vi "上下管柱装配.vi"() -> ()   [LabVIEW 2018]
uses:
  <vilib>/Utility/config.llb/NI_LVConfig.lvlib
  Global_Variable/Global.vi
  Global_Variable/Global1.vi
  Global_Variable/A131258.vi
  <vilib>/addons/database/NI_Database_API.lvlib
  <vilib>/addons/database/Connection.llb/Conn Execute.vi
  <vilib>/addons/database/Recordset.llb/Rec Fetch Recordset Data (R).vi
  <vilib>/addons/database/Connection.llb/DB Tools Open Connec (String).vi
panel:
  out "RIGHTMIN压力":string
  out "RIGHTMAX压力":string
  out "RIGHT位移":string
  out "LEFTMIN压力":string
  out "LEFTMAX压力":string
  out "LEFT位移":string
  out "RESULT":string
  out "PRODUCTID":string
  out "USERID":string
  out "上管柱码":string
  out "产品型号":string
  in  "附加信息 3":string
  in  "设备状态 3":enum16{"设备离线", "设备正常", "设备缺料", "设备故障", "质量报警"}(ring)=enum."质量报警"
  in  "附加信息 2":string
  in  "设备状态 2":enum16{"设备离线", "设备正常", "设备缺料", "设备故障", "质量报警"}(ring)=enum."设备缺料"
  in  "质量报警":bool
  in  "设备缺料":bool
  in  "附加信息":string
  in  "设备状态":enum16{"设备离线", "设备正常", "设备缺料", "设备故障", "质量报警"}(ring)=enum."设备故障"
  in  "设备故障":bool
  out "前序deviceID":string
  out "deviceID":string
  out "CODE_ID":string
  out "联机模式":string
  out "用户权限":string
  out "用户名":string
  in  "报表":string[][](table)=[["mm"], ["mm/s"]]
  in  "判定结果 3":bool[][](array[boolean])=[[TRUE]]
  in  "选项卡控件 2":enum32{"左工位压装曲线", "右工位压装曲线 ", "参数查看"}(tab)
  out "左压装下限":dbl format="%#.2f"
  out "左压装上限":dbl format="%#.2f"
  out "左下限2":dbl format="%#.2f"
  out "左上限2":dbl format="%#.2f"
  out "左下限1":dbl format="%#.2f"
  out "左上限1":dbl format="%#.2f"
  out "压装最大位移(mm)":dbl
  out "判定结果":bool
  out "力位移曲线":cluster{dbl[], dbl[]}[](graph)
  out "位移区间最大压力(KN)":dbl
  out "位移区间最小压力(KN)":dbl
  out "右位移下限":dbl format="%#.2f"
  out "右位移上限":dbl format="%#.2f"
  out "右下限2":dbl format="%#.2f"
  out "右上限2":dbl format="%#.2f"
  out "右下限1":dbl format="%#.2f"
  out "右上限1":dbl format="%#.2f"
  out "压装最大位移(mm) 2":dbl
  out "判定结果 2":bool
  out "力位移曲线 2":cluster{dbl[], dbl[]}[](graph)
  out "位移区间最大压力(KN) 2":dbl
  out "位移区间最小压力(KN) 2":dbl
  in  "删除":bool
  in  "确定":bool
  in  "添加":bool
  in  "退出":bool
  in  "更新":bool
  in  "产品型号":string(combo)
  in  "选项卡控件 3":enum32{"左工位参数", "右工位参数", "产品管理", "用户管理"}(tab)
  in  "左工位坐标轴参数":string[][](table)=[["mm"], ["mm/s"]]
  in  "左工位判定框参数":string[][](table)=[["mm"], ["mm/s"]]
  in  "左工位结果判定参数":string[][](table)=[["mm"], ["mm/s"]]
  in  "右工位结果判定参数":string[][](table)=[["mm"], ["mm/s"]]
  in  "右工位判定框参数":string[][](table)=[["mm"], ["mm/s"]]
  in  "右工位坐标轴参数":string[][](table)=[["mm"], ["mm/s"]]
  in  "请输入添加的产品名称":string
  in  "请选择要删除的产品":string(combo)
  in  "确定按钮":bool
  # "180上下柱管总成装配"
  # "上限"
  # "下限"
  # "上限"
  # "下限"
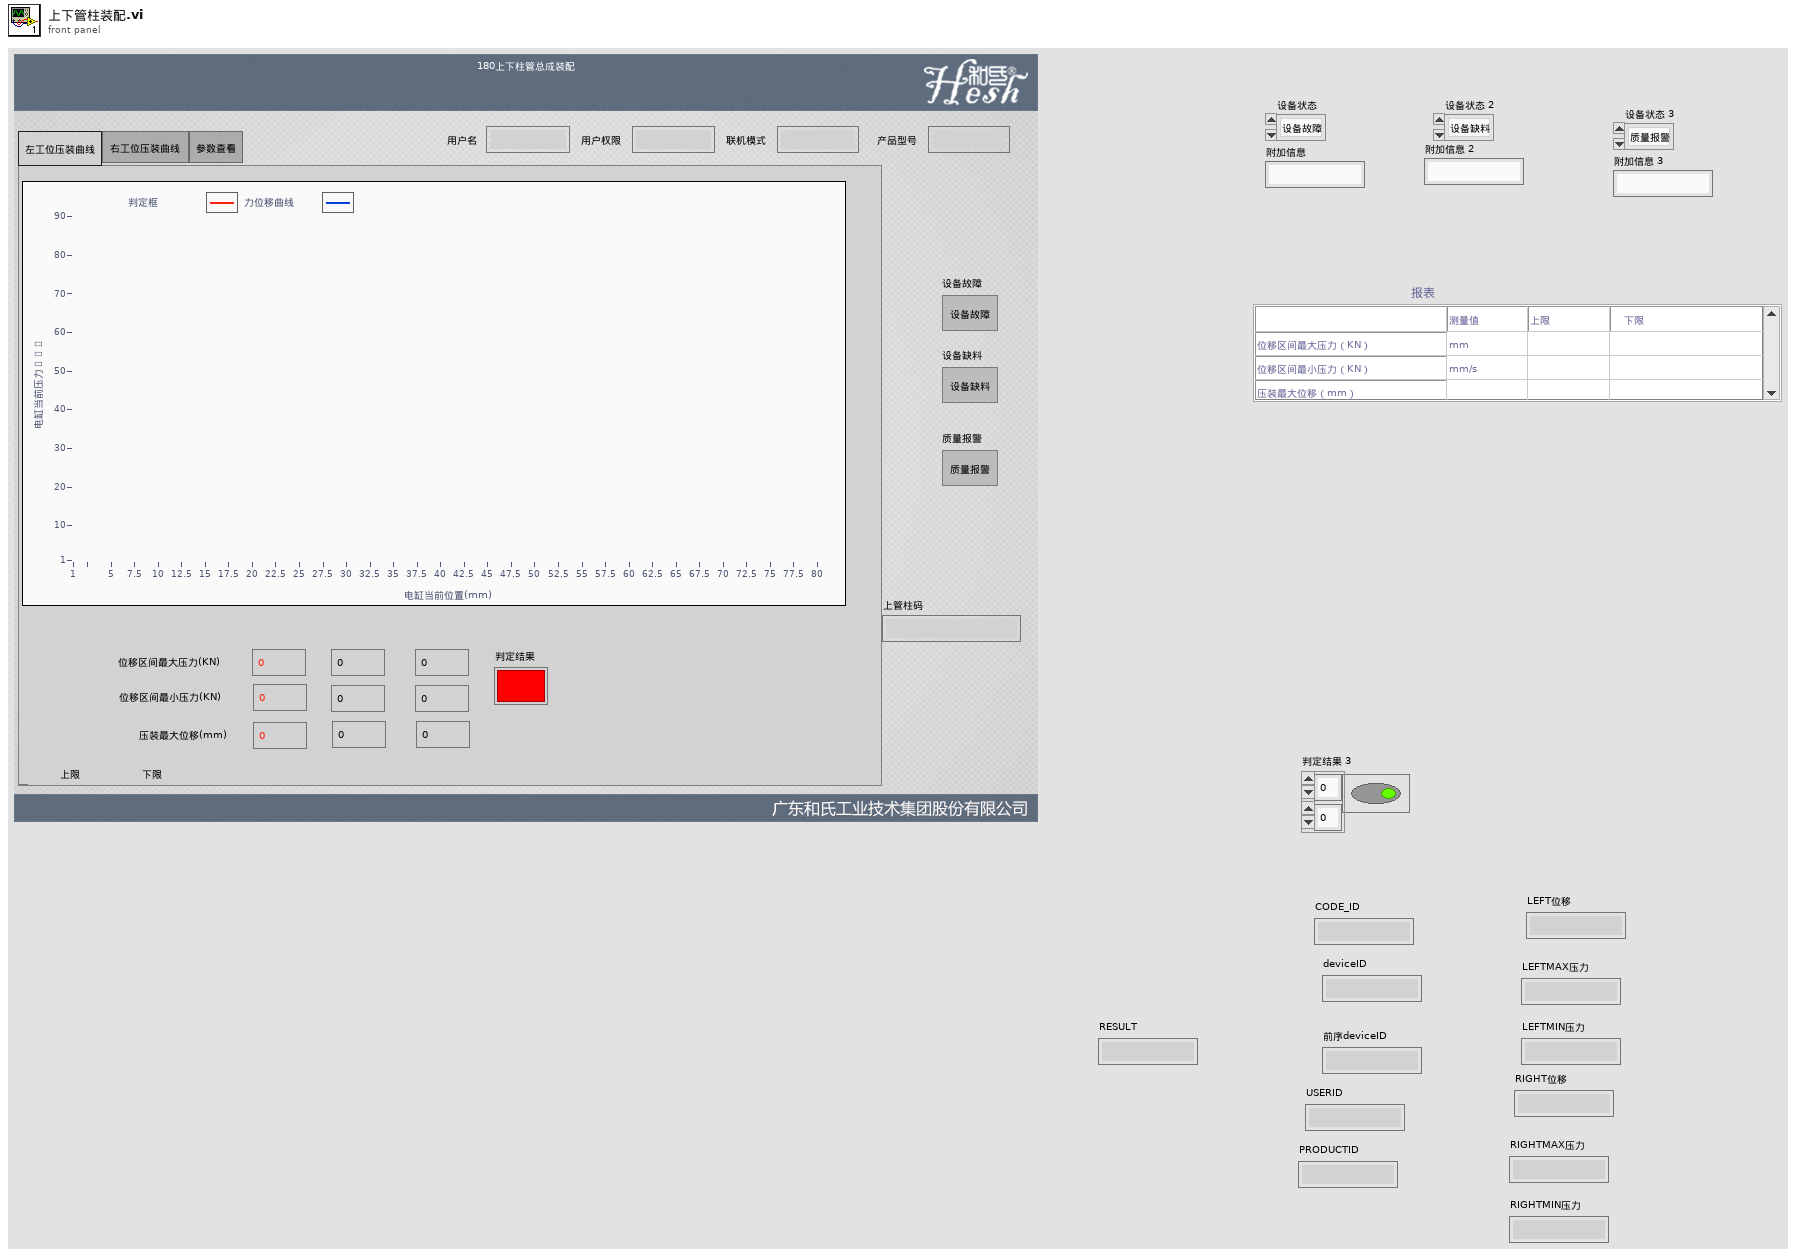
[diagram p1: front panel]
types:
  T1 = enum32{"Invalid", "Standard", "Closed", "Hidden", "Minimized", "Maximized"}
  T2 = cluster{"设备名称":string, "用户名":void, "设备状态":enum16{"设备离线", "设备正常", "设备缺料", "设备故障", "质量报警"}, "附加信息":string}
  T3 = typedef "NI_LVConfig.lvlib/Config Data RefNum.ctl" = refnum<k1>
  T4 = cluster{i64, i64, "table":string, "位移区间最小压力(KN) 2":dbl, "右下限2":dbl, "右上限2":dbl, "table":string, "RIGHTMIN压力":string}
  T5 = cluster{i64, i64, "table":string, "压装最大位移(mm) 2":dbl, "右位移下限":dbl, "右位移上限":dbl, "table":string, "RIGHT位移":string}
  T6 = cluster{i64, i64, "table":string, "位移区间最大压力(KN) 2":dbl, "右下限1":dbl, "右上限1":dbl, "table":string, "RIGHTMAX压力":string}
  T7 = cluster{i64, i64, "table":string, "位移区间最小压力(KN) 2":dbl, "右下限2":dbl, "右上限2":dbl, "table":string, "RIGHTMIN压力":string}[]
  T8 = typedef "NI_Database_API.lvlib/Conn ObjectReference.ctl" = refnum<k1>
  T9 = cluster{i64, i64, "位移区间最小压力(KN) 2":dbl, "右下限2":dbl, "右上限2":dbl, "table":string, "RIGHTMIN压力":string}
  T10 = cluster{i64, i64, i64, "RESULT":string, "result string":string}
  T11 = cluster{i64, i64, i64, "RESULT":string, "result string":string}[]
  T12 = typedef "NI_Database_API.lvlib/Rec ObjectReference.ctl" = refnum<k1>
  T13 = cluster{"设备名称":string, "用户名":void, "设备状态 2":enum16{"设备离线", "设备正常", "设备缺料", "设备故障", "质量报警"}, "附加信息 2":string}
  T14 = cluster{"设备名称":string, "用户名":void, "设备状态 3":enum16{"设备离线", "设备正常", "设备缺料", "设备故障", "质量报警"}, "附加信息 3":string}
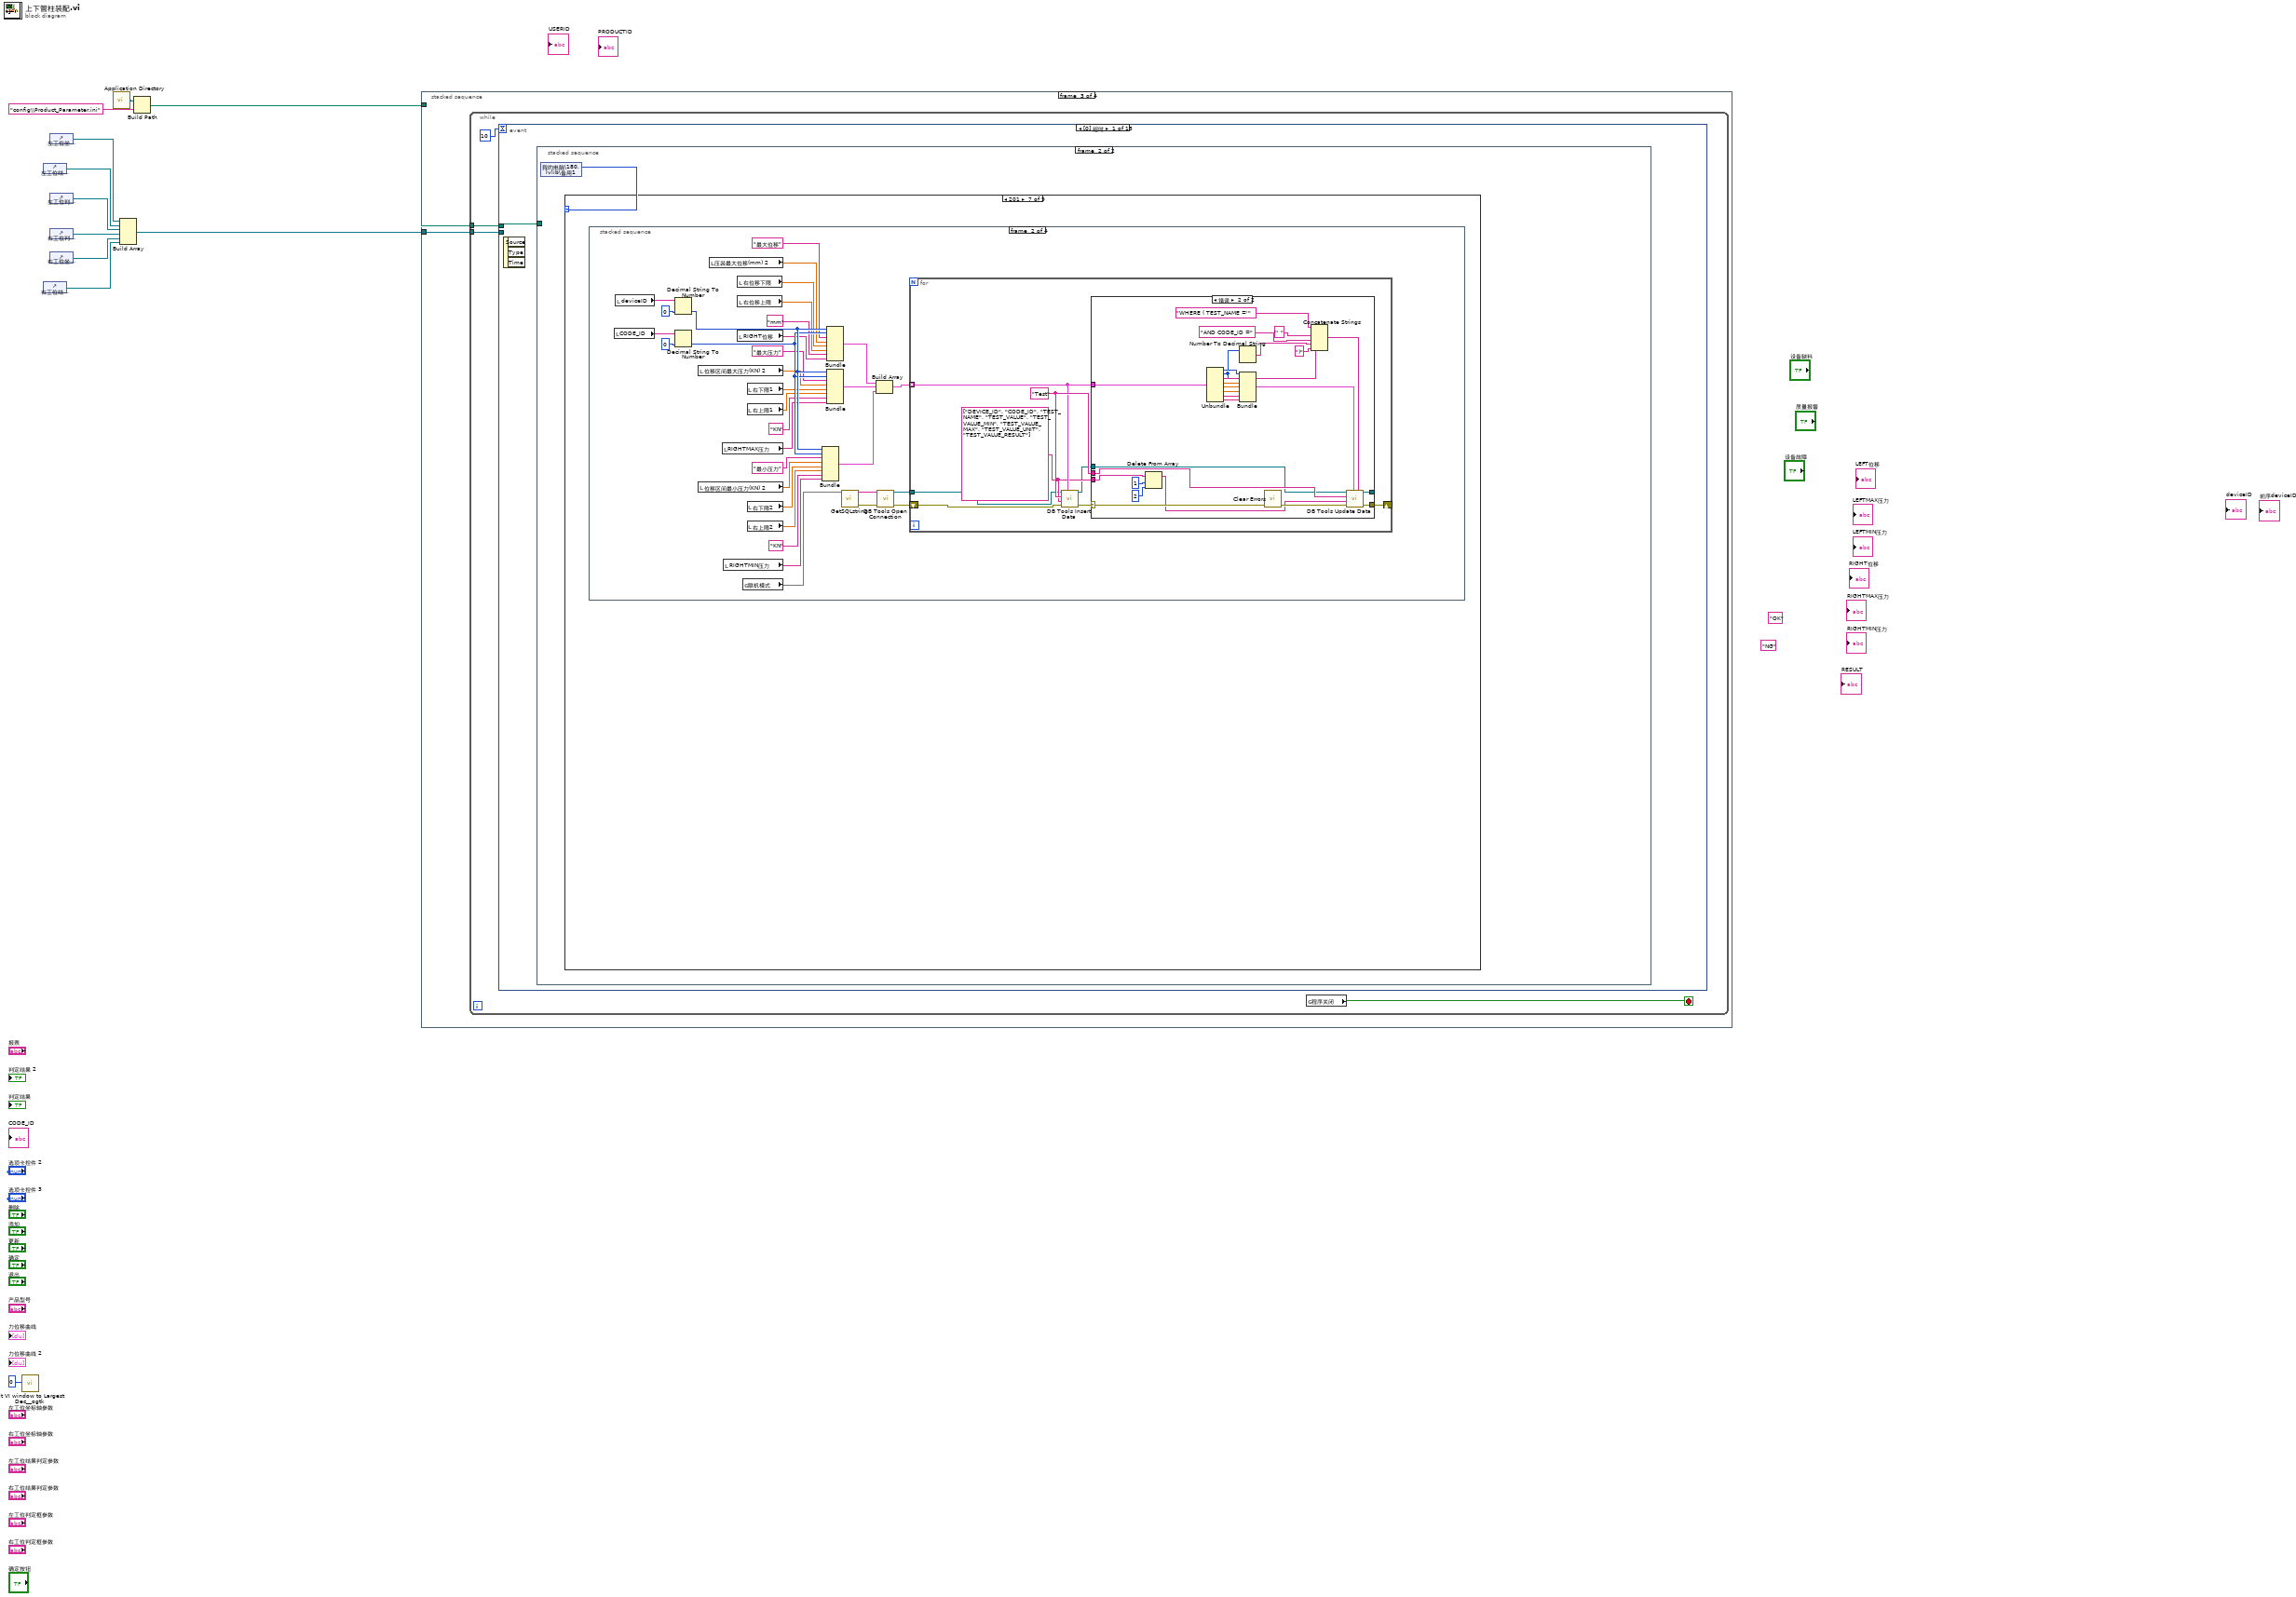
[diagram p0: block diagram]
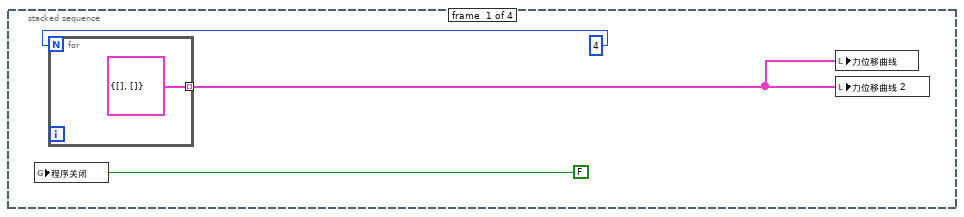
[diagram p2: hidden frame]
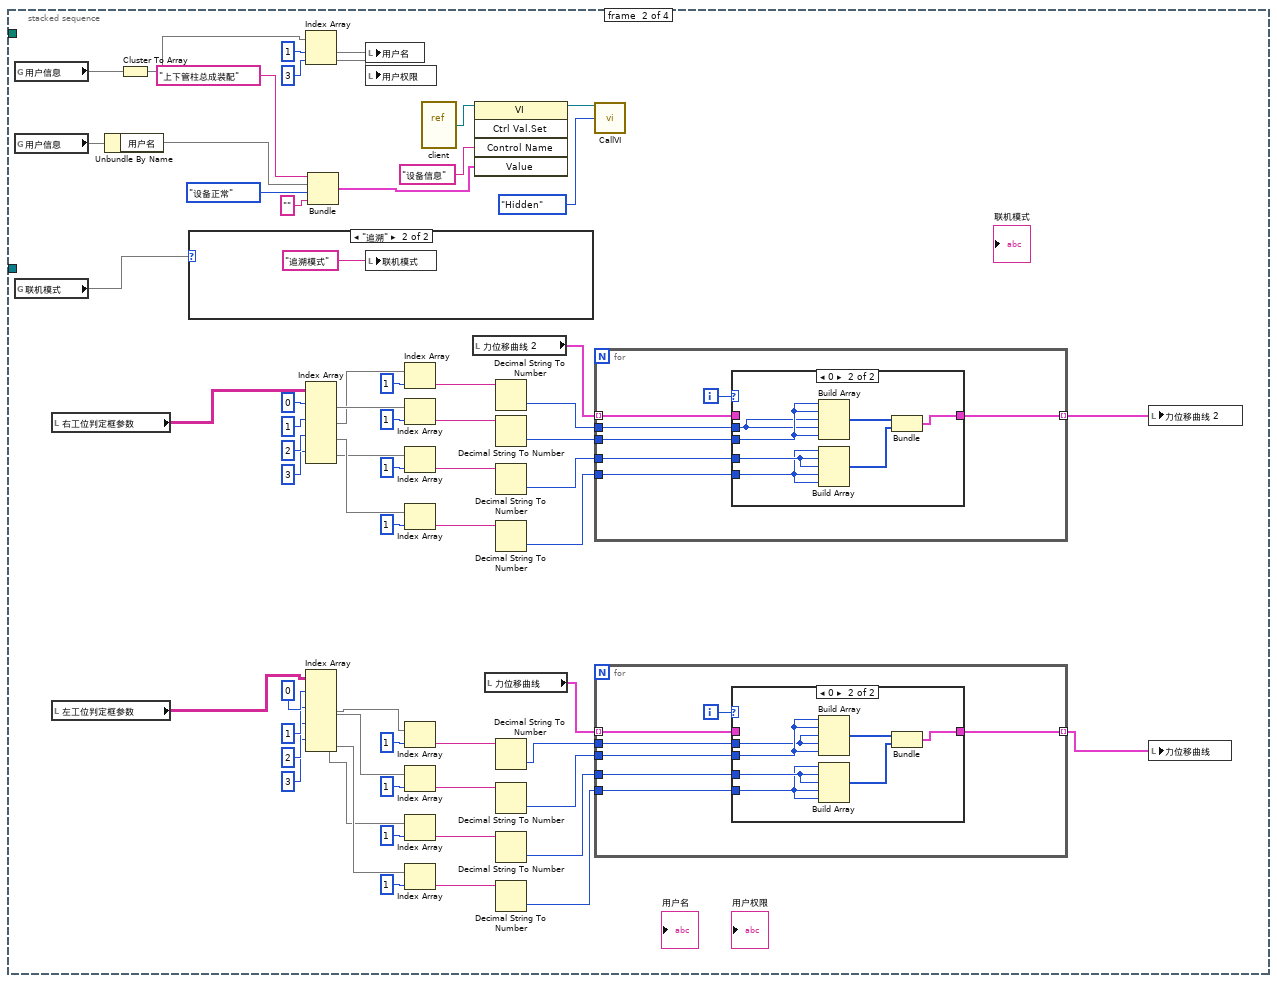
[diagram p3: hidden frame]
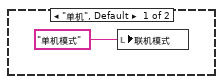
[diagram p4: hidden frame]
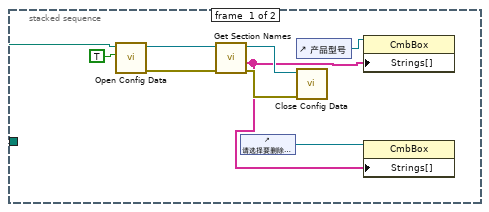
[diagram p7: hidden frame]
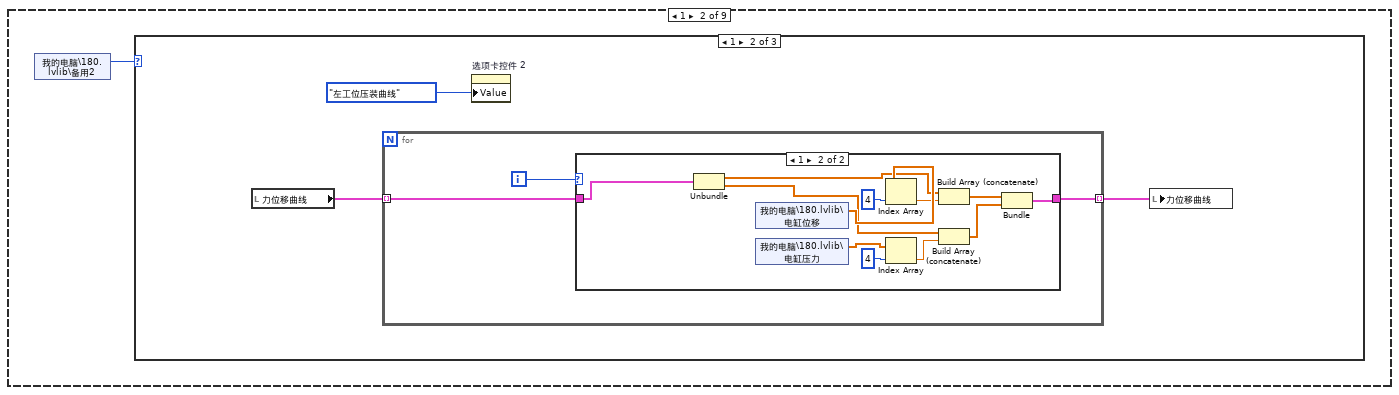
[diagram p9: hidden frame]
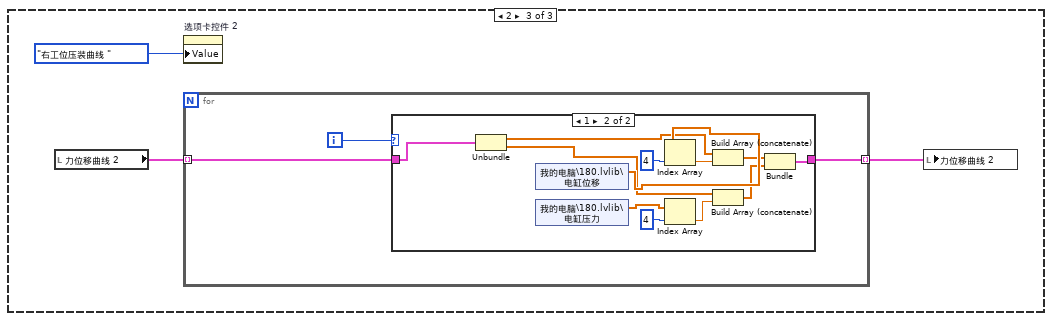
[diagram p12: hidden frame]
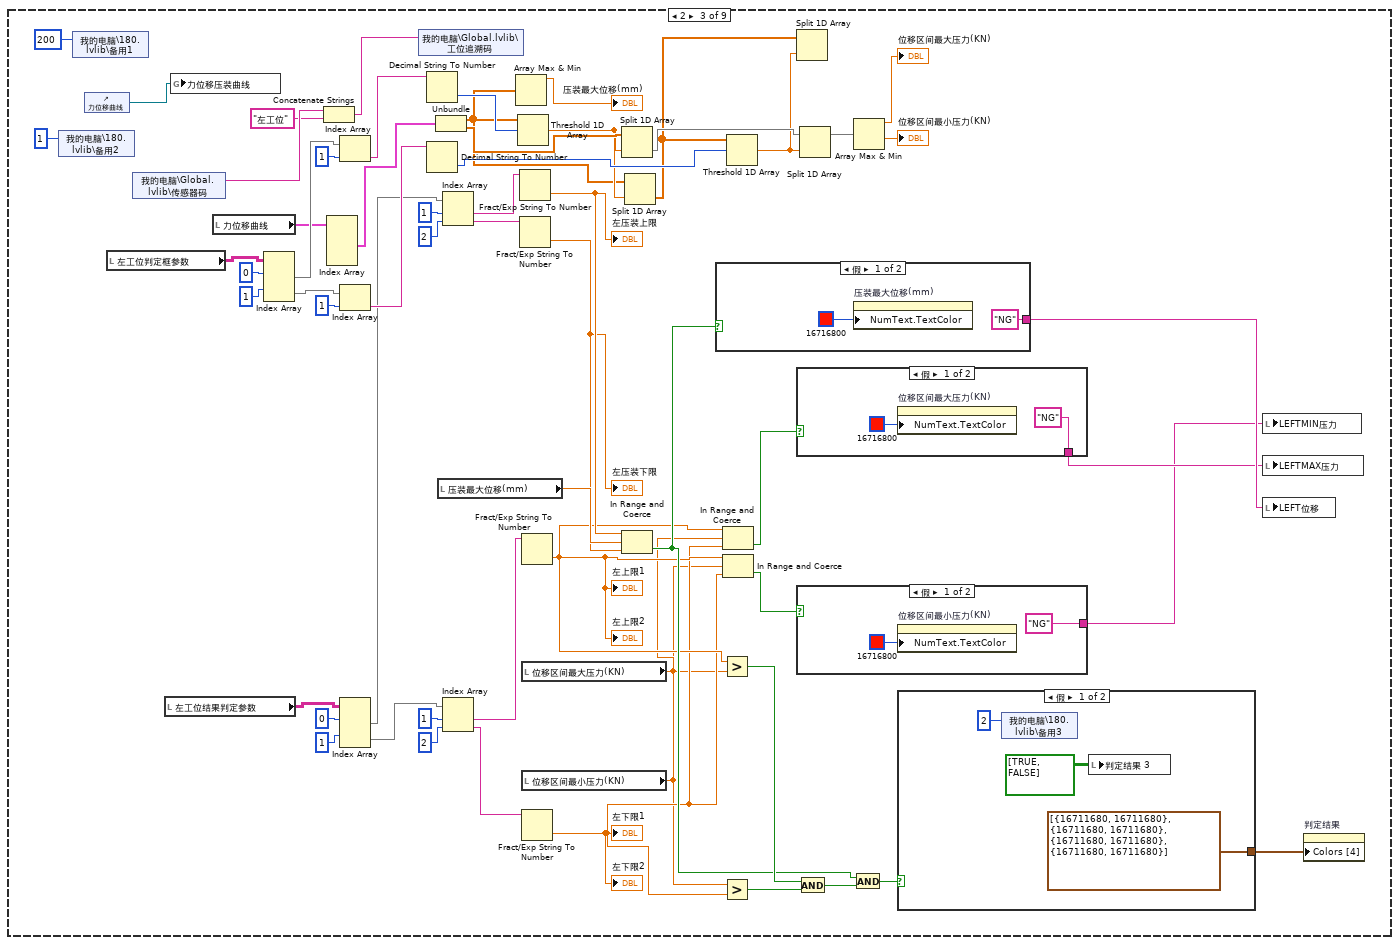
[diagram p14: hidden frame]
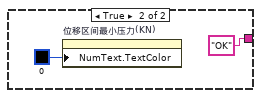
[diagram p15: hidden frame]
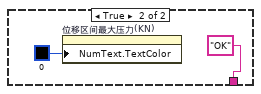
[diagram p16: hidden frame]
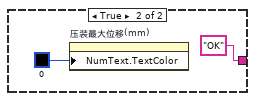
[diagram p17: hidden frame]
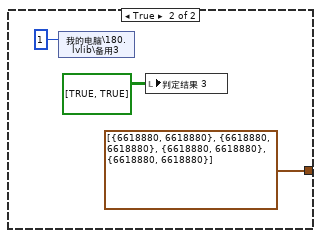
[diagram p18: hidden frame]
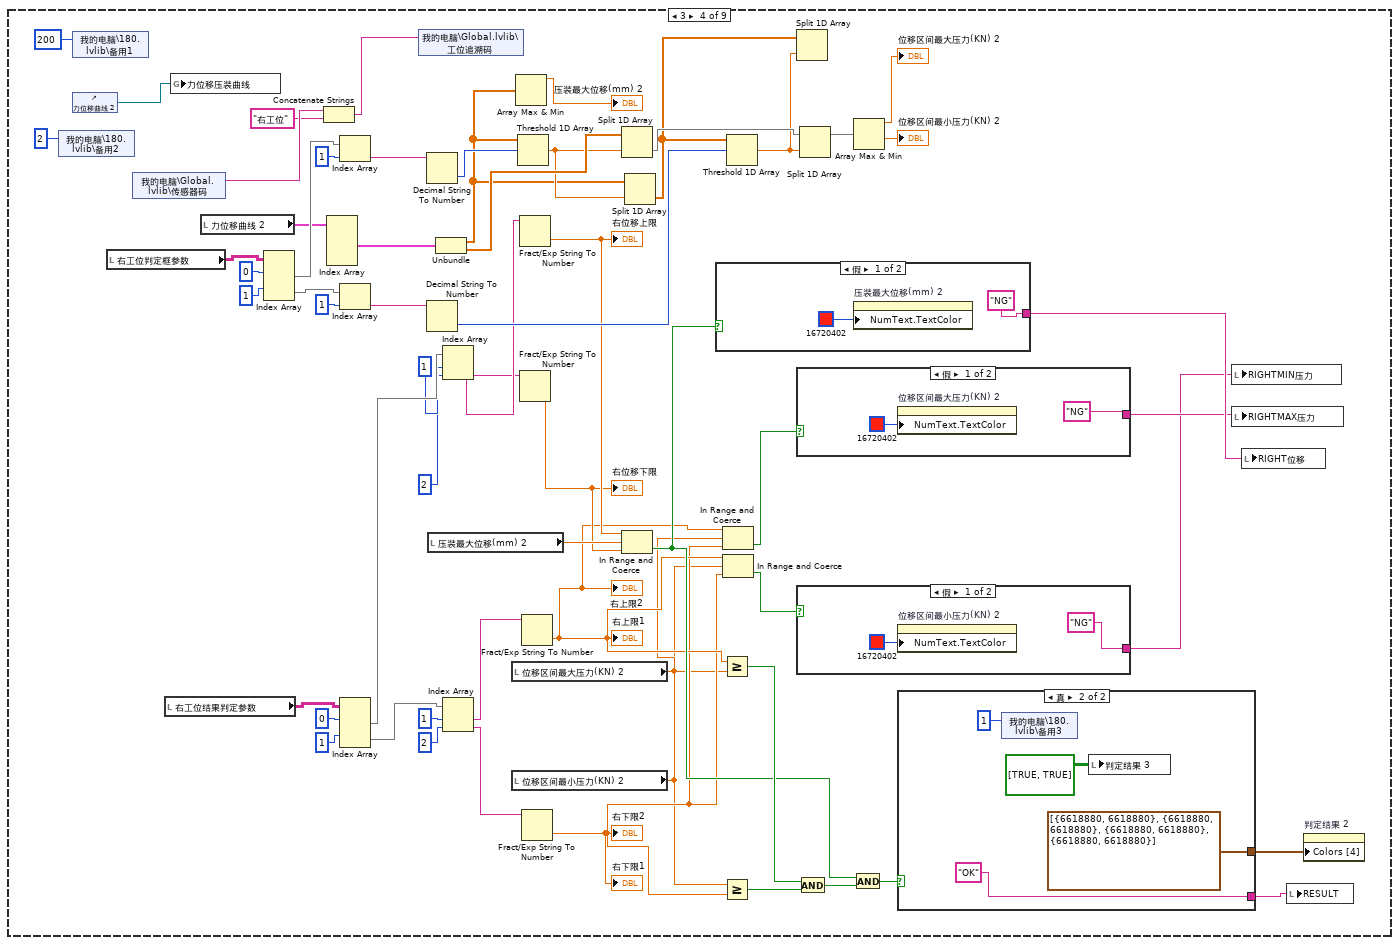
[diagram p19: hidden frame]
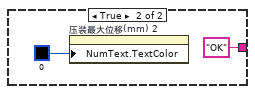
[diagram p20: hidden frame]
diagram:
  (unwired) "NG" ("RESULT")
  (unwired) "OK" ("RESULT")
  n1 = call <userlib>:"Fit VI window to Largest Dec__ogtk.vi"("border spacing (2 px)"=0) -> ()  [unwired: 5 in, 2 out]
  n2 = control-ref of="左工位结果判定参数"() -> (w5:refnum<vi>)
  n3 = control-ref of="右工位结果判定参数"() -> (w1:refnum<vi>)
  n4 = control-ref of="左工位坐标轴参数"() -> (w6:refnum<vi>)
  n5 = control-ref of="左工位判定框参数"() -> (w4:refnum<vi>)
  n6 = control-ref of="右工位判定框参数"() -> (w3:refnum<vi>)
  n7 = control-ref of="右工位坐标轴参数"() -> (w2:refnum<vi>)
  n8 = call <vilib>:"Application Directory.vi"() -> ("Application Directory"=w11:path)
  n9 = Build Array(w6, w5, w4, w3, w2, w1) -> (w7:refnum<vi>[])
  n10 = Build Path(base path=w11, name or relative path="config\\Product_Parameter.ini" ("名称或相对路径")) -> (appended path=w8:path)
  n11 = stacked-sequence {
    tunnel: w8 -> [_ _ w112 _]
    tunnel: w7 -> [_ _ w111 _]
    frame #0 {
      n12 = global write "Global.vi" "程序关闭"(FALSE ("程序关闭")) -> ()
      n13 = for {
        N: 4 -> [_]
        tunnel: [cluster{dbl[], dbl[]} {[], []}] -> w13 mode=indexing
      }
      n14 = local write "力位移曲线"(w13) -> ()
      n15 = local write "力位移曲线 2"(w13) -> ()
    }
    frame #1 {
      n16 = global read "Global1.vi" "用户信息"() -> (w32)
      n17 = global read "Global1.vi" "用户信息"() -> (w23)
      n18 = global read "Global1.vi" "联机模式"() -> (w26)
      n19 = local read "右工位判定框参数"() -> (w36:string[][])
      n20 = local read "左工位判定框参数"() -> (w33:string[][])
      n21 = Unbundle By Name(w23) -> ("用户名"=w22)
      n22 = Cluster To Array(cluster=w32) -> (array=w31:void[])
      n23 = case shown="\"追溯\"" w26 {
        frame "单机", Default {
          n24 = local write "联机模式"("单机模式" ("联机模式")) -> ()
        }
        frame "追溯" {
          n25 = local write "联机模式"("追溯模式" ("联机模式")) -> ()
        }
      }
      n26 = Index Array(array=w31, index #1=1 ("索引"), index #2=3 ("索引")) -> (element #1=w28, element #2=w27)
      n27 = Index Array(array=w36, index (row) #1=0 ("索引 (行)"), index (row) #2=1 ("索引 (行)"), index (row) #3=2 ("索引 (行)"), index (row) #4=3 ("索引 (行)")) -> (element #1=w52:string[], element #2=w47:string[], element #3=w46:string[], element #4=w45:string[])  [unwired: 4 in]
      n28 = Index Array(array=w33, index (row) #1=0 ("索引 (行)"), index (row) #2=1 ("索引 (行)"), index (row) #3=2 ("索引 (行)"), index (row) #4=3 ("索引 (行)")) -> (element #1=w74:string[], element #2=w69:string[], element #3=w68:string[], element #4=w67:string[])  [unwired: 4 in]
      n29 = Bundle("设备名称"="上下管柱总成装配", "用户名"=w22, "设备状态"=enum16{"设备离线", "设备正常", "设备缺料", "设备故障", "质量报警"}."设备正常", "附加信息"="") -> (w21:T2)  [unwired: 1 in]
      n30 = local write "用户名"(w28) -> ()
      n31 = local write "用户权限"(w27) -> ()
      n32 = Index Array(array=w47, index=1 ("索引")) -> (element=w39:string)
      n33 = Index Array(array=w52, index=1 ("索引")) -> (element=w40:string)
      n34 = Index Array(array=w45, index=1 ("索引")) -> (element=w37:string)
      n35 = Index Array(array=w46, index=1 ("索引")) -> (element=w38:string)
      n36 = Index Array(array=w69, index=1 ("索引")) -> (element=w61:string)
      n37 = Index Array(array=w74, index=1 ("索引")) -> (element=w62:string)
      n38 = Index Array(array=w67, index=1 ("索引")) -> (element=w59:string)
      n39 = Index Array(array=w68, index=1 ("索引")) -> (element=w60:string)
      n40 = vi-ref "client.vi"() -> (w25:refnum<vi>)
      n41 = local read "力位移曲线 2"() -> (w35:cluster{dbl[], dbl[]}[])
      n42 = invoke class="VI" method="Ctrl Val.Set"(reference=w25, "Control Name"="设备信息" ("控件名"), "Value"=w21) -> (reference out=w24:refnum<vi>)  [unwired: 2 in, 4 out]
      n43 = local read "力位移曲线"() -> (w57:cluster{dbl[], dbl[]}[])
      n44 = Decimal String To Number(string=w39) -> (number=w43:i32)  [unwired: 2 in, 1 out]
      n45 = Decimal String To Number(string=w40) -> (number=w44:i32)  [unwired: 2 in, 1 out]
      n46 = Decimal String To Number(string=w37) -> (number=w42:i32)  [unwired: 2 in, 1 out]
      n47 = Decimal String To Number(string=w38) -> (number=w41:i32)  [unwired: 2 in, 1 out]
      n48 = Decimal String To Number(string=w61) -> (number=w65:i32)  [unwired: 2 in, 1 out]
      n49 = Decimal String To Number(string=w62) -> (number=w66:i32)  [unwired: 2 in, 1 out]
      n50 = Decimal String To Number(string=w59) -> (number=w64:i32)  [unwired: 2 in, 1 out]
      n51 = Decimal String To Number(string=w60) -> (number=w63:i32)  [unwired: 2 in, 1 out]
      n52 = call "CallVI.vi"("VI引用"=w24, "状态"=T1."Hidden") -> ()  [unwired: 11 in, 3 out]
      n53 = for {
        tunnel: [w87] -> w34 mode=indexing
        tunnel: w35 -> [w86] mode=indexing
        tunnel: w44 -> [w84]
        tunnel: w43 -> [w83]
        tunnel: w42 -> [w82]
        tunnel: w41 -> [w81]
        i -> [w85]
        n54 = case shown="0" w85 {
          tunnel: [w88 w93] -> w87
          tunnel: w86 -> [w88 _]
          tunnel: w84 -> [_ w92]
          tunnel: w83 -> [_ w91]
          tunnel: w82 -> [_ w90]
          tunnel: w81 -> [_ w89]
          frame Default {
          }
          frame 0 {
            n55 = Build Array(w92, w92, w91, w91, w92) -> (w94:i32[])
            n56 = Build Array(w89, w90, w90, w89, w89) -> (w95:i32[])
            n57 = Bundle(w94, w95) -> (w93:cluster{i32[], i32[]})  [unwired: 1 in]
          }
        }
      }
      n58 = for {
        tunnel: [w102] -> w58 mode=indexing
        tunnel: w57 -> [w101] mode=indexing
        tunnel: w66 -> [w99]
        tunnel: w65 -> [w98]
        tunnel: w64 -> [w97]
        tunnel: w63 -> [w96]
        i -> [w100]
        n59 = case shown="0" w100 {
          tunnel: [w103 w108] -> w102
          tunnel: w101 -> [w103 _]
          tunnel: w99 -> [_ w107]
          tunnel: w98 -> [_ w106]
          tunnel: w97 -> [_ w105]
          tunnel: w96 -> [_ w104]
          frame Default {
          }
          frame 0 {
            n60 = Build Array(w107, w107, w106, w106, w107) -> (w109:i32[])
            n61 = Build Array(w104, w105, w105, w104, w104) -> (w110:i32[])
            n62 = Bundle(w109, w110) -> (w108:cluster{i32[], i32[]})  [unwired: 1 in]
          }
        }
      }
      n63 = local write "力位移曲线 2"(w34) -> ()
      n64 = local write "力位移曲线"(w58) -> ()
    }
    frame #2 {
      n65 = while {
        tunnel: w112 -> [w115]
        tunnel: w111 -> [w114]
        stop <- w113 stop-if-true
        n66 = event shown="[0] 超时" {
          selector: _ -> [_ _ _ _ _ _ _ _ _ _ _ _ _]
          dyn-events: _ -> [_ _ _ _ _ _ _ _ _ _ _ _ _]
          timeout: 10 -> [_ _ _ _ _ _ _ _ _ _ _ _ _]
          tunnel: w115 -> [w117 w648 _ w816 w835 _ w850 _ _ _ _ _ _]
          tunnel: w114 -> [_ _ _ w815 w834 _ w849 _ _ _ _ _ _]
          event Timeout {
            n67 = event-data() -> ()  [unwired: 1 in, 3 out]
            n68 = stacked-sequence {
              tunnel: w117 -> [w118 _]
              frame #0 {
                n69 = call <vilib>:"Open Config Data.vi"("create file if necessary (T)"=TRUE, "configuration file path"=w118) -> ("error out"=w123:errorcluster, "refnum"=w122:T3)  [unwired: 7 in, 1 out]
                n70 = call <vilib>:"Get Section Names.vi"("error in (no error)"=w123, "refnum"=w122) -> ("error out"=w125:errorcluster, "section names"=w121:string[], "refnum out"=w124:T3)  [unwired: 7 in]
                n71 = control-ref of="请选择要删除的产品"() -> (w119:refnum<vi>)
                n72 = control-ref of="产品型号"() -> (w120:refnum<vi>)
                n73 = call <vilib>:"Close Config Data.vi"("error in (no error)"=w125, "refnum"=w124) -> ()  [unwired: 8 in, 2 out]
                n74 = property on="属性节点" class="CmbBox"(reference=w120, "Strings[]"=w121) -> ()  [unwired: 1 in, 2 out]
                n75 = property on="属性节点" class="CmbBox"(reference=w119, "Strings[]"=w121) -> ()  [unwired: 1 in, 2 out]
              }
              frame #1 {
                n76 = shared-variable "我的电脑\\180.lvlib\\备用1"() -> (w127:u16)  [unwired: 1 in, 1 out]
                n77 = case shown="201" w127 {
                  frame 0, Default {
                  }
                  frame 1 {
                    n78 = shared-variable "我的电脑\\180.lvlib\\备用2"() -> (w128:u16)  [unwired: 1 in, 1 out]
                    n79 = case shown="1" w128 {
                      frame 0, Default {
                      }
                      frame 1 {
                        n80 = local read "力位移曲线"() -> (w130:cluster{dbl[], dbl[]}[])
                        n81 = for {
                          tunnel: [w134] -> w129 mode=indexing
                          tunnel: w130 -> [w133] mode=indexing
                          i -> [w132]
                          n82 = case shown="1" w132 {
                            tunnel: [w135 w139] -> w134
                            tunnel: w133 -> [w135 w138]
                            frame Default {
                            }
                            frame 1 {
                              n83 = Unbundle(w138) -> (w143:dbl[], w142:dbl[])
                              n84 = shared-variable "我的电脑\\180.lvlib\\电缸位移"() -> (w145:sgl[])  [unwired: 1 in, 1 out]
                              n85 = shared-variable "我的电脑\\180.lvlib\\电缸压力"() -> (w147:sgl[])  [unwired: 1 in, 1 out]
                              n86 = Index Array(array=w145, index=4) -> (element=w136:sgl)
                              n87 = Index Array(array=w147, index=4) -> (element=w137:sgl)
                              n88 = Build Array (concatenate)(w143, w136) -> (w141:dbl[])
                              n89 = Build Array (concatenate)(w142, w137) -> (w140:dbl[])
                              n90 = Bundle(w141, w140) -> (w139:cluster{dbl[], dbl[]})  [unwired: 1 in]
                            }
                          }
                        }
                        n91 = property on="选项卡控件 2" class="TabCtl (严格)"("Value"=enum32{"左工位压装曲线", "右工位压装曲线 ", "参数查看"}."左工位压装曲线" ("选项卡控件 2")) -> ()  [unwired: 2 in, 2 out]
                        n92 = local write "力位移曲线"(w129) -> ()
                      }
                      frame 2 {
                        n93 = local read "力位移曲线 2"() -> (w149:cluster{dbl[], dbl[]}[])
                        n94 = property on="选项卡控件 2" class="TabCtl (严格)"("Value"=enum32{"左工位压装曲线", "右工位压装曲线 ", "参数查看"}."右工位压装曲线 " ("选项卡控件 2")) -> ()  [unwired: 2 in, 2 out]
                        n95 = for {
                          tunnel: [w153] -> w150 mode=indexing
                          tunnel: w149 -> [w152] mode=indexing
                          i -> [w151]
                          n96 = case shown="1" w151 {
                            tunnel: [w154 w158] -> w153
                            tunnel: w152 -> [w154 w157]
                            frame Default {
                            }
                            frame 1 {
                              n97 = Unbundle(w157) -> (w162:dbl[], w161:dbl[])
                              n98 = shared-variable "我的电脑\\180.lvlib\\电缸位移"() -> (w164:sgl[])  [unwired: 1 in, 1 out]
                              n99 = shared-variable "我的电脑\\180.lvlib\\电缸压力"() -> (w166:sgl[])  [unwired: 1 in, 1 out]
                              n100 = Index Array(array=w164, index=4) -> (element=w155:sgl)
                              n101 = Index Array(array=w166, index=4) -> (element=w156:sgl)
                              n102 = Build Array (concatenate)(w162, w155) -> (w160:dbl[])
                              n103 = Build Array (concatenate)(w161, w156) -> (w159:dbl[])
                              n104 = Bundle(w160, w159) -> (w158:cluster{dbl[], dbl[]})  [unwired: 1 in]
                            }
                          }
                        }
                        n105 = local write "力位移曲线 2"(w150) -> ()
                      }
                    }
                  }
                  frame 2 {
                    n106 = shared-variable "我的电脑\\180.lvlib\\备用2"(u16 1 ("备用1")) -> ()  [unwired: 1 in, 1 out]
                    n107 = shared-variable "我的电脑\\180.lvlib\\备用1"(u16 200 ("备用1")) -> ()  [unwired: 1 in, 1 out]
                    n108 = control-ref of="力位移曲线"() -> (w175:refnum<vi>)
                    n109 = local read "左工位判定框参数"() -> (w225:string[][])
                    n110 = shared-variable "我的电脑\\Global.lvlib\\传感器码"() -> (w173:string)  [unwired: 1 in, 1 out]
                    n111 = local read "左工位结果判定参数"() -> (w197:string[][])
                    n112 = global write "A131258.vi" "力位移压装曲线"(w175) -> ()
                    n113 = local read "力位移曲线"() -> (w220:cluster{dbl[], dbl[]}[])
                    n114 = Index Array(array=w225, index (row) #1=0 ("索引 (行)"), index (row) #2=1 ("索引 (行)")) -> (element #1=w221:string[], element #2=w222:string[])  [unwired: 2 in]
                    n115 = Concatenate Strings(w173, "左工位" ("字符串")) -> (w174:string)
                    n116 = Index Array(array=w220) -> (element #2=w219:cluster{dbl[], dbl[]})  [unwired: 4 in, 3 out]
                    n117 = Index Array(array=w221, index=1 ("索引")) -> (element=w223:string)
                    n118 = Index Array(array=w222, index=1 ("索引")) -> (element=w224:string)
                    n119 = Index Array(array=w197, index (row) #1=0 ("索引 (行)"), index (row) #2=1 ("索引 (行)")) -> (element #1=w198:string[], element #2=w203:string[])  [unwired: 2 in]
                    n120 = shared-variable "我的电脑\\Global.lvlib\\工位追溯码"(w174) -> ()  [unwired: 1 in, 1 out]
                    n121 = Decimal String To Number(string=w223) -> (number=w206:i32)  [unwired: 2 in, 1 out]
                    n122 = Decimal String To Number(string=w224) -> (number=w226:i32)  [unwired: 2 in, 1 out]
                    n123 = Unbundle(w219) -> (w204:dbl[], w218:dbl[])
                    n124 = local read "压装最大位移(mm)"() -> (w194:dbl)
                    n125 = Index Array(array=w198, index #1=1 ("索引"), index #2=2 ("索引")) -> (element #1=w193:string, element #2=w192:string)
                    n126 = Index Array(array=w203, index #1=1 ("索引"), index #2=2 ("索引")) -> (element #1=w191:string, element #2=w190:string)
                    n127 = Array Max & Min(array=w204) -> (max value=→"压装最大位移(mm)":dbl)  [unwired: 3 out]
                    n128 = Threshold 1D Array(2:w206, 3:w204) -> (0:w217:dbl)  [unwired: 1 in]
                    n129 = Fract/Exp String To Number(string=w193) -> (number=w184:dbl)  [unwired: 3 in, 1 out]
                    "左压装上限" <- w184
                    n130 = Fract/Exp String To Number(string=w192) -> (number=w183:dbl)  [unwired: 3 in, 1 out]
                    "左压装下限" <- w183
                    n131 = Fract/Exp String To Number(string=w191) -> (number=w179:dbl)  [unwired: 3 in, 1 out]
                    "左上限1" <- w179
                    "左上限2" <- w179
                    n132 = local read "位移区间最大压力(KN)"() -> (w177:dbl)
                    n133 = local read "位移区间最小压力(KN)"() -> (w176:dbl)
                    n134 = Fract/Exp String To Number(string=w190) -> (number=w178:dbl)  [unwired: 3 in, 1 out]
                    "左下限1" <- w178
                    "左下限2" <- w178
                    n135 = Split 1D Array(array=w218, index=w217) -> (second subarray=w216:dbl[])  [unwired: 1 out]
                    n136 = In Range and Coerce(upper limit=w184, x=w194, lower limit=w183) -> (In Range?=w182:bool)  [unwired: 1 out]
                    n137 = Split 1D Array(array=w204, index=w217) -> (second subarray=w215:dbl[])  [unwired: 1 out]
                    n138 = case shown="假" w182 {
                      tunnel: ["NG" ("RESULT") "OK" ("RESULT")] -> w169
                      frame False {
                        n139 = property on="压装最大位移(mm)" class="DigNum (严格)"("NumText.TextColor"=u32 16716800) -> ()  [unwired: 2 in, 2 out]
                      }
                      frame True {
                        n140 = property on="压装最大位移(mm)" class="DigNum (严格)"("NumText.TextColor"=u32 0) -> ()  [unwired: 2 in, 2 out]
                      }
                    }
                    n141 = Greater?(x=w179, y=w177) -> (0:w189:bool)
                    n142 = Greater?(x=w176, y=w178) -> (0:w188:bool)
                    n143 = In Range and Coerce(upper limit=w179, x=w177, lower limit=w178) -> (In Range?=w181:bool)  [unwired: 1 out]
                    n144 = In Range and Coerce(upper limit=w179, x=w176, lower limit=w178) -> (In Range?=w180:bool)  [unwired: 1 out]
                    n145 = Threshold 1D Array(2:w226, 3:w215) -> (0:w214:dbl)  [unwired: 1 in]
                    n146 = Split 1D Array(array=w215, index=w214) -> ()  [unwired: 2 out]
                    n147 = case shown="假" w181 {
                      tunnel: ["NG" ("RESULT") "OK" ("RESULT")] -> w168
                      frame False {
                        n148 = property on="位移区间最大压力(KN)" class="DigNum (严格)"("NumText.TextColor"=u32 16716800) -> ()  [unwired: 2 in, 2 out]
                      }
                      frame True {
                        n149 = property on="位移区间最大压力(KN)" class="DigNum (严格)"("NumText.TextColor"=u32 0) -> ()  [unwired: 2 in, 2 out]
                      }
                    }
                    n150 = case shown="假" w180 {
                      tunnel: ["NG" ("RESULT") "OK" ("RESULT")] -> w167
                      frame False {
                        n151 = property on="位移区间最小压力(KN)" class="DigNum (严格)"("NumText.TextColor"=u32 16716800) -> ()  [unwired: 2 in, 2 out]
                      }
                      frame True {
                        n152 = property on="位移区间最小压力(KN)" class="DigNum (严格)"("NumText.TextColor"=u32 0) -> ()  [unwired: 2 in, 2 out]
                      }
                    }
                    n153 = And(x=w189, y=w188) -> (x .and. y?=w187:bool)
                    n154 = Split 1D Array(array=w216, index=w214) -> (first subarray=w213:dbl[])  [unwired: 1 out]
                    n155 = And(x=w182, y=w187) -> (x .and. y?=w186:bool)
                    n156 = Array Max & Min(array=w213) -> (max value=→"位移区间最大压力(KN)":dbl, min value=→"位移区间最小压力(KN)":dbl)  [unwired: 2 out]
                    n157 = case shown="假" w186 {
                      tunnel: [cluster{u32, u32}[] [{16711680, 16711680}, {16711680, 16711680}, {16711680, 16711680}, {16711680, 16711680}] cluster{u32, u32}[] [{6618880, 6618880}, {6618880, 6618880}, {6618880, 6618880}, {6618880, 6618880}]] -> w185
                      frame False {
                        n158 = shared-variable "我的电脑\\180.lvlib\\备用3"(u16 2 ("备用1")) -> ()  [unwired: 1 in, 1 out]
                        n159 = local write "判定结果 3"(bool[][] [[TRUE, FALSE]] ("判定结果")) -> ()
                      }
                      frame True {
                        n160 = shared-variable "我的电脑\\180.lvlib\\备用3"(u16 1 ("备用1")) -> ()  [unwired: 1 in, 1 out]
                        n161 = local write "判定结果 3"(bool[][] [[TRUE, TRUE]] ("判定结果")) -> ()
                      }
                    }
                    n162 = local write "LEFTMIN压力"(w167) -> ()
                    n163 = local write "LEFTMAX压力"(w168) -> ()
                    n164 = local write "LEFT位移"(w169) -> ()
                    n165 = property on="判定结果" class="Bool (严格)"("Colors [4]"=w185) -> ()  [unwired: 2 in, 2 out]
                  }
                  frame 3 {
                    n166 = shared-variable "我的电脑\\180.lvlib\\备用2"(u16 2 ("备用1")) -> ()  [unwired: 1 in, 1 out]
                    n167 = shared-variable "我的电脑\\180.lvlib\\备用1"(u16 200 ("备用1")) -> ()  [unwired: 1 in, 1 out]
                    n168 = control-ref of="力位移曲线 2"() -> (w254:refnum<vi>)
                    n169 = local read "右工位判定框参数"() -> (w291:string[][])
                    n170 = shared-variable "我的电脑\\Global.lvlib\\传感器码"() -> (w252:string)  [unwired: 1 in, 1 out]
                    n171 = local read "右工位结果判定参数"() -> (w284:string[][])
                    n172 = global write "A131258.vi" "力位移压装曲线"(w254) -> ()
                    n173 = local read "力位移曲线 2"() -> (w292:cluster{dbl[], dbl[]}[])
                    n174 = Index Array(array=w291, index (row) #1=0 ("索引 (行)"), index (row) #2=1 ("索引 (行)")) -> (element #1=w301:string[], element #2=w302:string[])  [unwired: 2 in]
                    n175 = Concatenate Strings(w252, "右工位" ("字符串")) -> (w253:string)
                    n176 = Index Array(array=w292) -> (element #2=w300:cluster{dbl[], dbl[]})  [unwired: 4 in, 3 out]
                    n177 = Index Array(array=w301, index=1 ("索引")) -> (element=w303:string)
                    n178 = Index Array(array=w302, index=1 ("索引")) -> (element=w304:string)
                    n179 = Index Array(array=w284, index (row) #1=0 ("索引 (行)"), index (row) #2=1 ("索引 (行)")) -> (element #1=w285:string[], element #2=w286:string[])  [unwired: 2 in]
                    n180 = shared-variable "我的电脑\\Global.lvlib\\工位追溯码"(w253) -> ()  [unwired: 1 in, 1 out]
                    n181 = Decimal String To Number(string=w303) -> (number=w289:i32)  [unwired: 2 in, 1 out]
                    n182 = Decimal String To Number(string=w304) -> (number=w305:i32)  [unwired: 2 in, 1 out]
                    n183 = local read "压装最大位移(mm) 2"() -> (w279:dbl)
                    n184 = Unbundle(w300) -> (w287:dbl[], w299:dbl[])
                    n185 = Index Array(array=w285, index #1=1 ("索引"), index #2=2 ("索引")) -> (element #1=w283:string, element #2=w280:string)
                    n186 = Index Array(array=w286, index #1=1 ("索引"), index #2=2 ("索引")) -> (element #1=w282:string, element #2=w281:string)
                    n187 = local read "位移区间最大压力(KN) 2"() -> (w266:dbl)
                    n188 = local read "位移区间最小压力(KN) 2"() -> (w265:dbl)
                    n189 = Array Max & Min(array=w287) -> (max value=→"压装最大位移(mm) 2":dbl)  [unwired: 3 out]
                    n190 = Threshold 1D Array(2:w289, 3:w287) -> (0:w290:dbl)  [unwired: 1 in]
                    n191 = Fract/Exp String To Number(string=w283) -> (number=w274:dbl)  [unwired: 3 in, 1 out]
                    "右位移上限" <- w274
                    n192 = Fract/Exp String To Number(string=w280) -> (number=w273:dbl)  [unwired: 3 in, 1 out]
                    "右位移下限" <- w273
                    n193 = Fract/Exp String To Number(string=w282) -> (number=w268:dbl)  [unwired: 3 in, 1 out]
                    "右上限1" <- w268
                    "右上限2" <- w268
                    n194 = Fract/Exp String To Number(string=w281) -> (number=w267:dbl)  [unwired: 3 in, 1 out]
                    "右下限1" <- w267
                    "右下限2" <- w267
                    n195 = Split 1D Array(array=w299, index=w290) -> (second subarray=w298:dbl[])  [unwired: 1 out]
                    n196 = In Range and Coerce(upper limit=w274, x=w279, lower limit=w273) -> (In Range?=w271:bool)  [unwired: 1 out]
                    n197 = Split 1D Array(array=w287, index=w290) -> (second subarray=w297:dbl[])  [unwired: 1 out]
                    n198 = case shown="假" w271 {
                      tunnel: ["NG" ("RESULT") "OK" ("RESULT")] -> w247
                      frame False {
                        n199 = property on="压装最大位移(mm) 2" class="DigNum (严格)"("NumText.TextColor"=u32 16720402) -> ()  [unwired: 2 in, 2 out]
                      }
                      frame True {
                        n200 = property on="压装最大位移(mm) 2" class="DigNum (严格)"("NumText.TextColor"=u32 0) -> ()  [unwired: 2 in, 2 out]
                      }
                    }
                    n201 = Greater Or Equal?(x=w268, y=w266) -> (x >= y?=w272:bool)
                    n202 = Greater Or Equal?(x=w265, y=w267) -> (x >= y?=w277:bool)
                    n203 = In Range and Coerce(upper limit=w268, x=w266, lower limit=w267) -> (In Range?=w269:bool)  [unwired: 1 out]
                    n204 = In Range and Coerce(upper limit=w268, x=w265, lower limit=w267) -> (In Range?=w270:bool)  [unwired: 1 out]
                    n205 = Threshold 1D Array(2:w305, 3:w297) -> (0:w296:dbl)  [unwired: 1 in]
                    n206 = Split 1D Array(array=w297, index=w296) -> ()  [unwired: 2 out]
                    n207 = case shown="假" w269 {
                      tunnel: ["NG" ("RESULT") "OK" ("RESULT")] -> w246
                      frame False {
                        n208 = property on="位移区间最大压力(KN) 2" class="DigNum (严格)"("NumText.TextColor"=u32 16720402) -> ()  [unwired: 2 in, 2 out]
                      }
                      frame True {
                        n209 = property on="位移区间最大压力(KN) 2" class="DigNum (严格)"("NumText.TextColor"=u32 0) -> ()  [unwired: 2 in, 2 out]
                      }
                    }
                    n210 = case shown="假" w270 {
                      tunnel: ["NG" ("RESULT") "OK" ("RESULT")] -> w245
                      frame False {
                        n211 = property on="位移区间最小压力(KN) 2" class="DigNum (严格)"("NumText.TextColor"=u32 16720402) -> ()  [unwired: 2 in, 2 out]
                      }
                      frame True {
                        n212 = property on="位移区间最小压力(KN) 2" class="DigNum (严格)"("NumText.TextColor"=u32 0) -> ()  [unwired: 2 in, 2 out]
                      }
                    }
                    n213 = And(x=w272, y=w277) -> (x .and. y?=w278:bool)
                    n214 = Split 1D Array(array=w298, index=w296) -> (first subarray=w295:dbl[])  [unwired: 1 out]
                    n215 = And(x=w271, y=w278) -> (x .and. y?=w276:bool)
                    n216 = Array Max & Min(array=w295) -> (max value=→"位移区间最大压力(KN) 2":dbl, min value=→"位移区间最小压力(KN) 2":dbl)  [unwired: 2 out]
                    n217 = case shown="真" w276 {
                      tunnel: [cluster{u32, u32}[] [{16711680, 16711680}, {16711680, 16711680}, {16711680, 16711680}, {16711680, 16711680}] cluster{u32, u32}[] [{6618880, 6618880}, {6618880, 6618880}, {6618880, 6618880}, {6618880, 6618880}]] -> w275
                      tunnel: ["NG" ("RESULT") "OK" ("RESULT")] -> w248
                      frame False {
                        n218 = shared-variable "我的电脑\\180.lvlib\\备用3"(u16 2 ("备用1")) -> ()  [unwired: 1 in, 1 out]
                        n219 = local write "判定结果 3"(bool[][] [[TRUE, FALSE]] ("判定结果")) -> ()
                      }
                      frame True {
                        n220 = shared-variable "我的电脑\\180.lvlib\\备用3"(u16 1 ("备用1")) -> ()  [unwired: 1 in, 1 out]
                        n221 = local write "判定结果 3"(bool[][] [[TRUE, TRUE]] ("判定结果")) -> ()
                      }
                    }
                    n222 = local write "RIGHTMIN压力"(w245) -> ()
                    n223 = local write "RIGHTMAX压力"(w246) -> ()
                    n224 = local write "RIGHT位移"(w247) -> ()
                    n225 = local write "RESULT"(w248) -> ()
                    n226 = property on="判定结果 2" class="Bool (严格)"("Colors [4]"=w275) -> ()  [unwired: 2 in, 2 out]
                  }
                  frame 100 {
                    n227 = stacked-sequence {
                      frame #0 {
                        w328 = cluster{u32, u32}[] [{12369084, 12369084}, {12369084, 12369084}, {12369084, 12369084}, {12369084, 12369084}]
                        w329 = u32 0
                        w330 = 0.0 ("压装最大位移(mm)")
                        n228 = global read "Global.vi" "Result"() -> (w326:refnum<vi>)
                        n229 = local write "压装最大位移(mm)"(w330) -> ()
                        n230 = local write "位移区间最小压力(KN)"(w330) -> ()
                        n231 = local write "位移区间最大压力(KN)"(w330) -> ()
                        n232 = local write "压装最大位移(mm) 2"(w330) -> ()
                        n233 = local write "位移区间最小压力(KN) 2"(w330) -> ()
                        n234 = local write "位移区间最大压力(KN) 2"(w330) -> ()
                        n235 = property on="位移区间最大压力(KN) 2" class="DigNum (严格)"("NumText.TextColor"=w329) -> ()  [unwired: 2 in, 2 out]
                        n236 = property on="位移区间最小压力(KN) 2" class="DigNum (严格)"("NumText.TextColor"=w329) -> ()  [unwired: 2 in, 2 out]
                        n237 = property on="压装最大位移(mm) 2" class="DigNum (严格)"("NumText.TextColor"=w329) -> ()  [unwired: 2 in, 2 out]
                        n238 = property on="位移区间最大压力(KN)" class="DigNum (严格)"("NumText.TextColor"=w329) -> ()  [unwired: 2 in, 2 out]
                        n239 = property on="位移区间最小压力(KN)" class="DigNum (严格)"("NumText.TextColor"=w329) -> ()  [unwired: 2 in, 2 out]
                        n240 = property on="压装最大位移(mm)" class="DigNum (严格)"("NumText.TextColor"=w329) -> ()  [unwired: 2 in, 2 out]
                        n241 = for {
                          N: 4 -> [_]
                          tunnel: [cluster{dbl[], dbl[]} {[], []}] -> w331 mode=indexing
                        }
                        n242 = property class="Tbl"(reference=w326, "Value"=string[][] []) -> ()  [unwired: 1 in, 2 out]
                        n243 = local write "力位移曲线 2"(w331) -> ()
                        n244 = local write "力位移曲线"(w331) -> ()
                        n245 = property on="判定结果" class="Bool (严格)"("Colors [4]"=w328) -> ()  [unwired: 2 in, 2 out]
                        n246 = property on="判定结果 2" class="Bool (严格)"("Colors [4]"=w328) -> ()  [unwired: 2 in, 2 out]
                      }
                      frame #1 {
                        n247 = local read "左工位判定框参数"() -> (w335:string[][])
                        n248 = Index Array(array=w335, index (row) #1=0 ("索引 (行)"), index (row) #2=1 ("索引 (行)"), index (row) #3=2 ("索引 (行)"), index (row) #4=3 ("索引 (行)")) -> (element #1=w352:string[], element #2=w347:string[], element #3=w346:string[], element #4=w345:string[])  [unwired: 4 in]
                        n249 = Index Array(array=w347, index=1 ("索引")) -> (element=w339:string)
                        n250 = Index Array(array=w352, index=1 ("索引")) -> (element=w340:string)
                        n251 = Index Array(array=w345, index=1 ("索引")) -> (element=w337:string)
                        n252 = Index Array(array=w346, index=1 ("索引")) -> (element=w338:string)
                        n253 = local read "力位移曲线"() -> (w336:cluster{dbl[], dbl[]}[])
                        n254 = Fract/Exp String To Number(string=w339) -> (number=w343:dbl)  [unwired: 3 in, 1 out]
                        n255 = Fract/Exp String To Number(string=w340) -> (number=w344:dbl)  [unwired: 3 in, 1 out]
                        n256 = Fract/Exp String To Number(string=w337) -> (number=w342:dbl)  [unwired: 3 in, 1 out]
                        n257 = Fract/Exp String To Number(string=w338) -> (number=w341:dbl)  [unwired: 3 in, 1 out]
                        n258 = for {
                          tunnel: [w363] -> w334 mode=indexing
                          tunnel: w336 -> [w362] mode=indexing
                          tunnel: w344 -> [w360]
                          tunnel: w343 -> [w359]
                          tunnel: w342 -> [w358]
                          tunnel: w341 -> [w357]
                          i -> [w361]
                          n259 = case shown="0" w361 {
                            tunnel: [w364 w369] -> w363
                            tunnel: w362 -> [w364 _]
                            tunnel: w360 -> [_ w368]
                            tunnel: w359 -> [_ w367]
                            tunnel: w358 -> [_ w366]
                            tunnel: w357 -> [_ w365]
                            frame Default {
                            }
                            frame 0 {
                              n260 = Build Array(w368, w368, w367, w367, w368) -> (w370:dbl[])
                              n261 = Build Array(w365, w366, w366, w365, w365) -> (w371:dbl[])
                              n262 = Bundle(w370, w371) -> (w369:cluster{dbl[], dbl[]})  [unwired: 1 in]
                            }
                          }
                        }
                        n263 = local write "力位移曲线"(w334) -> ()
                      }
                      frame #2 {
                        n264 = local read "右工位判定框参数"() -> (w372:string[][])
                        n265 = Index Array(array=w372, index (row) #1=0 ("索引 (行)"), index (row) #2=1 ("索引 (行)"), index (row) #3=2 ("索引 (行)"), index (row) #4=3 ("索引 (行)")) -> (element #1=w390:string[], element #2=w385:string[], element #3=w384:string[], element #4=w383:string[])  [unwired: 4 in]
                        n266 = Index Array(array=w385, index=1 ("索引")) -> (element=w377:string)
                        n267 = Index Array(array=w390, index=1 ("索引")) -> (element=w378:string)
                        n268 = Index Array(array=w383, index=1 ("索引")) -> (element=w375:string)
                        n269 = Index Array(array=w384, index=1 ("索引")) -> (element=w376:string)
                        n270 = local read "力位移曲线 2"() -> (w374:cluster{dbl[], dbl[]}[])
                        n271 = Fract/Exp String To Number(string=w377) -> (number=w381:dbl)  [unwired: 3 in, 1 out]
                        n272 = Fract/Exp String To Number(string=w378) -> (number=w382:dbl)  [unwired: 3 in, 1 out]
                        n273 = Fract/Exp String To Number(string=w375) -> (number=w380:dbl)  [unwired: 3 in, 1 out]
                        n274 = Fract/Exp String To Number(string=w376) -> (number=w379:dbl)  [unwired: 3 in, 1 out]
                        n275 = for {
                          tunnel: [w401] -> w373 mode=indexing
                          tunnel: w374 -> [w400] mode=indexing
                          tunnel: w382 -> [w398]
                          tunnel: w381 -> [w397]
                          tunnel: w380 -> [w396]
                          tunnel: w379 -> [w395]
                          i -> [w399]
                          n276 = case shown="0" w399 {
                            tunnel: [w402 w407] -> w401
                            tunnel: w400 -> [w402 _]
                            tunnel: w398 -> [_ w406]
                            tunnel: w397 -> [_ w405]
                            tunnel: w396 -> [_ w404]
                            tunnel: w395 -> [_ w403]
                            frame Default {
                            }
                            frame 0 {
                              n277 = Build Array(w406, w406, w405, w405, w406) -> (w408:dbl[])
                              n278 = Build Array(w403, w404, w404, w403, w403) -> (w409:dbl[])
                              n279 = Bundle(w408, w409) -> (w407:cluster{dbl[], dbl[]})  [unwired: 1 in]
                            }
                          }
                        }
                        n280 = local write "力位移曲线 2"(w373) -> ()
                      }
                    }
                  }
                  frame 200 {
                    n281 = stacked-sequence {
                      frame #0 {
                        n282 = Wait (ms)(milliseconds to wait=u32 500 ("等待时间（毫秒）")) -> ()  [unwired: 1 out]
                        n283 = call "浮动通知.vi"("通知内容"="报表生成中" ("Status")) -> ()  [unwired: 11 in]
                      }
                      frame #1 {
                      }
                    }
                    n284 = control-ref of="报表"() -> (w410:refnum<vi>)
                    n285 = shared-variable "我的电脑\\180.lvlib\\备用2"() -> (w413:u16)  [unwired: 1 in, 1 out]
                    n286 = shared-variable "我的电脑\\180.lvlib\\备用1"(u16 201 ("备用1")) -> ()  [unwired: 1 in, 1 out]
                    n287 = global write "Global.vi" "Result"(w410) -> ()
                    n288 = case shown="1" w413 {
                      tunnel: [_ w414 w445] -> w411
                      frame 0, Default {
                      }
                      frame 1 {
                        n289 = local read "位移区间最大压力(KN)"() -> (w426:dbl)
                        n290 = local read "位移区间最小压力(KN)"() -> (w421:dbl)
                        n291 = local read "压装最大位移(mm)"() -> (w425:dbl)
                        n292 = local read "左压装上限"() -> (w418:dbl)
                        n293 = local read "左压装下限"() -> (w417:dbl)
                        n294 = local read "左上限1"() -> (w423:dbl)
                        n295 = local read "左下限1"() -> (w422:dbl)
                        n296 = local read "左上限2"() -> (w420:dbl)
                        n297 = local read "左下限2"() -> (w419:dbl)
                        n298 = Number To Fractional String(number=w426) -> (F-format string=w435:string)  [unwired: 3 in]
                        n299 = Number To Fractional String(number=w423) -> (F-format string=w434:string)  [unwired: 3 in]
                        n300 = Number To Fractional String(number=w422) -> (F-format string=w429:string)  [unwired: 3 in]
                        n301 = Number To Fractional String(number=w421) -> (F-format string=w432:string)  [unwired: 3 in]
                        n302 = Number To Fractional String(number=w420) -> (F-format string=w431:string)  [unwired: 3 in]
                        n303 = Number To Fractional String(number=w419) -> (F-format string=w428:string)  [unwired: 3 in]
                        n304 = Number To Fractional String(number=w425) -> (F-format string=w424:string)  [unwired: 3 in]
                        n305 = Number To Fractional String(number=w418) -> (F-format string=w416:string)  [unwired: 3 in]
                        n306 = Number To Fractional String(number=w417) -> (F-format string=w415:string)  [unwired: 3 in]
                        n307 = Build Array(w435, w434, w429) -> (w433:string[])
                        n308 = Build Array(w432, w431, w428) -> (w430:string[])
                        n309 = Build Array(w424, w416, w415) -> (w427:string[])
                        n310 = Build Array(w433, w430, w427) -> (w414:string[][])
                      }
                      frame 2 {
                        n311 = local read "位移区间最大压力(KN) 2"() -> (w444:dbl)
                        n312 = local read "位移区间最小压力(KN) 2"() -> (w441:dbl)
                        n313 = local read "压装最大位移(mm) 2"() -> (w438:dbl)
                        n314 = local read "右位移上限"() -> (w437:dbl)
                        n315 = local read "右位移下限"() -> (w436:dbl)
                        n316 = local read "右上限1"() -> (w443:dbl)
                        n317 = local read "右下限1"() -> (w442:dbl)
                        n318 = local read "右上限2"() -> (w440:dbl)
                        n319 = local read "右下限2"() -> (w439:dbl)
                        n320 = Number To Fractional String(number=w444) -> (F-format string=w457:string)  [unwired: 3 in]
                        n321 = Number To Fractional String(number=w443) -> (F-format string=w456:string)  [unwired: 3 in]
                        n322 = Number To Fractional String(number=w442) -> (F-format string=w451:string)  [unwired: 3 in]
                        n323 = Number To Fractional String(number=w441) -> (F-format string=w454:string)  [unwired: 3 in]
                        n324 = Number To Fractional String(number=w440) -> (F-format string=w453:string)  [unwired: 3 in]
                        n325 = Number To Fractional String(number=w439) -> (F-format string=w450:string)  [unwired: 3 in]
                        n326 = Number To Fractional String(number=w438) -> (F-format string=w448:string)  [unwired: 3 in]
                        n327 = Number To Fractional String(number=w437) -> (F-format string=w447:string)  [unwired: 3 in]
                        n328 = Number To Fractional String(number=w436) -> (F-format string=w446:string)  [unwired: 3 in]
                        n329 = Build Array(w457, w456, w451) -> (w455:string[])
                        n330 = Build Array(w454, w453, w450) -> (w452:string[])
                        n331 = Build Array(w448, w447, w446) -> (w449:string[])
                        n332 = Build Array(w455, w452, w449) -> (w445:string[][])
                      }
                    }
                    n333 = local write "报表"(w411) -> ()
                  }
                  frame 201 {
                    n334 = stacked-sequence {
                      frame #0 {
                        n335 = shared-variable "我的电脑\\Global.lvlib\\工位追溯码"() -> (w462:string)  [unwired: 1 in, 1 out]
                        n336 = call "Report_A131258.vi"("文件重命名"=TRUE, "文件名称"=w462, "布尔数组"="判定结果 3") -> ()  [unwired: 8 in, 1 out]
                        n337 = Wait (ms)(milliseconds to wait=u32 800 ("等待时间（毫秒）")) -> ()  [unwired: 1 out]
                      }
                      frame #1 {
                        n338 = local read "CODE_ID"() -> (w486:string)
                        n339 = local read "deviceID"() -> (w489:string)
                        n340 = Decimal String To Number(string=w489, default (0L)=i64 0 ("长度")) -> (number=w484:i64)  [unwired: 1 in, 1 out]
                        n341 = Decimal String To Number(string=w486, default (0L)=i64 0 ("长度")) -> (number=w483:i64)  [unwired: 1 in, 1 out]
                        n342 = local read "位移区间最大压力(KN) 2"() -> (w476:dbl)
                        n343 = local read "位移区间最小压力(KN) 2"() -> (w470:dbl)
                        n344 = local read "压装最大位移(mm) 2"() -> (w473:dbl)
                        n345 = local read "RIGHTMAX压力"() -> (w466:string)
                        n346 = local read "RIGHTMIN压力"() -> (w467:string)
                        n347 = local read "右位移下限"() -> (w472:dbl)
                        n348 = local read "右位移上限"() -> (w471:dbl)
                        n349 = local read "RIGHT位移"() -> (w465:string)
                        n350 = global read "Global1.vi" "联机模式"() -> (w490)
                        n351 = local read "右下限1"() -> (w475:dbl)
                        n352 = local read "右上限1"() -> (w474:dbl)
                        n353 = local read "右下限2"() -> (w469:dbl)
                        n354 = local read "右上限2"() -> (w468:dbl)
                        n355 = Bundle(w484, w483, "table"="最小压力", "位移区间最小压力(KN) 2"=w470, "右下限2"=w469, "右上限2"=w468, "table"="KN", "RIGHTMIN压力"=w467) -> (w464:T4)  [unwired: 1 in]
                        n356 = Bundle(w484, w483, "table"="最大位移", "压装最大位移(mm) 2"=w473, "右位移下限"=w472, "右位移上限"=w471, "table"="mm", "RIGHT位移"=w465) -> (w492:T5)  [unwired: 1 in]
                        n357 = Bundle(w484, w483, "table"="最大压力", "位移区间最大压力(KN) 2"=w476, "右下限1"=w475, "右上限1"=w474, "table"="KN", "RIGHTMAX压力"=w466) -> (w491:T6)  [unwired: 1 in]
                        n358 = call "GetSQLstring.vi"("联机模式"=w490) -> ("错误输出"=w494:errorcluster, "连接字符串"=w495:string)  [unwired: 9 in]
                        n359 = Build Array(w492, w491, w464) -> (w485:T7)
                        n360 = call-poly <vilib>:"DB Tools Open Connection.vi"("error in (no error)"=w494, "connection information"=w495) -> ("error out"=w496:errorcluster, "connection reference"=w493:T8)  [unwired: 6 in]
                        n361 = for {
                          tunnel: w485 -> [w501] mode=indexing
                          tunnel: w493 -> [w499]
                          shift-right: [w497] -> _
                          shift-left: w496 -> [w504]
                          w500 = string[] ["DEVICE_ID", "CODE_ID", "TEST_NAME", "TEST_VALUE", "TEST_VALUE_MIN", "TEST_VALUE_MAX", "TEST_VALUE_UNIT", "TEST_VALUE_RESULT"] ("columns")
                          w502 = "Test" ("table")
                          n362 = call <vilib>:"DB Tools Insert Data.vi"("data"=w501, "error in (no error)"=w504, "columns"=w500, "table"=w502, "connection reference"=w499) -> ("error out"=w503:errorcluster, "connection reference out"=w498:T8)  [unwired: 5 in]
                          n363 = case shown="错误" w503 {
                            selector: w503 -> [w505 w531]
                            tunnel: w500 -> [_ w528]
                            tunnel: w498 -> [w506 w513]
                            tunnel: w502 -> [_ w532]
                            tunnel: w501 -> [_ w522]
                            tunnel: [w506 w512] -> _
                            tunnel: [w505 w511] -> w497
                            frame No Error {
                            }
                            frame Error {
                              n364 = Delete From Array(array=w528, length=1 ("长度"), index=2 ("索引")) -> (array with subset deleted=w529:string[])  [unwired: 1 out]
                              n365 = Unbundle(w522) -> (w521:i64, w509:i64, "table"=w514:string, "位移区间最小压力(KN) 2"=w520:dbl, "右下限2"=w519:dbl, "右上限2"=w518:dbl, "table"=w517:string, "RIGHTMIN压力"=w516:string)
                              n366 = Number To Decimal String(number=w509) -> (decimal integer string=w508:string)  [unwired: 1 in]
                              n367 = Bundle(w521, w509, "位移区间最小压力(KN) 2"=w520, "右下限2"=w519, "右上限2"=w518, "table"=w517, "RIGHTMIN压力"=w516) -> (w515:T9)  [unwired: 1 in]
                              n368 = call <vilib>:"Clear Errors.vi"("error in (no error)"=w531) -> ("error out"=w530:errorcluster)  [unwired: 5 in, 1 out]
                              n369 = Concatenate Strings("WHERE ( TEST_NAME ='" ("condition"), w514, "' ", "AND CODE_ID =" ("condition"), w508, ")" ("condition")) -> (w524:string)
                              n370 = call <vilib>:"DB Tools Update Data.vi"("condition"=w524, "data"=w515, "error in (no error)"=w530, "columns"=w529, "table"=w532, "connection reference"=w513) -> ("error out"=w511:errorcluster, "connection reference out"=w512:T8)  [unwired: 4 in]
                            }
                          }
                        }
                      }
                      frame #2 {
                        n371 = Get Date/Time String(date format (0)=enum16{"short", "long", "abbreviated"}."short" ("日期格式(0)"), want seconds? (F)=FALSE ("需要秒？(F)")) -> (date string=w555:string, time string=w556:string)  [unwired: 1 in]
                        n372 = local read "RESULT"() -> (w534:string)
                        n373 = local read "CODE_ID"() -> (w553:string)
                        n374 = local read "deviceID"() -> (w551:string)
                        n375 = local read "USERID"() -> (w559:string)
                        n376 = Concatenate Strings(w555, " " ("字符串"), w556) -> (w558:string)
                        n377 = global read "Global1.vi" "联机模式"() -> (w533)
                        n378 = Decimal String To Number(string=w551, default (0L)=i64 0 ("默认(0 I32)")) -> (number=w552:i64)  [unwired: 1 in, 1 out]
                        n379 = Decimal String To Number(string=w559, default (0L)=i64 0 ("默认(0 I32)")) -> (number=w560:i64)  [unwired: 1 in, 1 out]
                        n380 = Decimal String To Number(string=w553, default (0L)=i64 0 ("默认(0 I32)")) -> (number=w554:i64)  [unwired: 1 in, 1 out]
                        n381 = Search and Replace String(replace all?=TRUE ("替换全部？(F)"), input string=w558, search string="/" ("替换字符串(\"\")"), replace string="-" ("替换字符串(\"\")")) -> (result string=w557:string)  [unwired: 4 in, 3 out]
                        n382 = Bundle(w552, w560, w554, "RESULT"=w534, "result string"=w557) -> (w549:T10)  [unwired: 1 in]
                        n383 = call "GetSQLstring.vi"("联机模式"=w533) -> ("错误输出"=w546:errorcluster, "连接字符串"=w545:string)  [unwired: 9 in]
                        n384 = Build Array(w549) -> (w550:T11)
                        n385 = call-poly <vilib>:"DB Tools Open Connection.vi"("error in (no error)"=w546, "connection information"=w545) -> ("error out"=w544:errorcluster, "connection reference"=w547:T8)  [unwired: 6 in]
                        n386 = for {
                          tunnel: w550 -> [w565] mode=indexing
                          tunnel: w547 -> [w563]
                          shift-right: [w561] -> w548
                          shift-left: w544 -> [w568]
                          w564 = string[] ["DEVICE_ID", "USER_ID", "CODE_ID", "RESULT_VALUE", "RESULT_TIME"] ("columns")
                          w566 = "Result" ("table")
                          n387 = call <vilib>:"DB Tools Insert Data.vi"("data"=w565, "error in (no error)"=w568, "columns"=w564, "table"=w566, "connection reference"=w563) -> ("error out"=w567:errorcluster, "connection reference out"=w562:T8)  [unwired: 5 in]
                          n388 = case shown="错误" w567 {
                            selector: w567 -> [w569 w590]
                            tunnel: w564 -> [_ w587]
                            tunnel: w562 -> [w570 w579]
                            tunnel: w566 -> [_ w591]
                            tunnel: w565 -> [_ w583]
                            tunnel: [w570 w578] -> _
                            tunnel: [w569 w577] -> w561
                            frame No Error {
                            }
                            frame Error {
                              n389 = Array Subset(array=w587, index=3 ("长度"), length=2 ("长度")) -> (w588:string[])
                              n390 = Unbundle(w583) -> (w572:i64, w575:i64, "RESULT"=w582:string, "result string"=w581:string)  [unwired: 1 out]
                              n391 = Number To Decimal String(number=w575) -> (decimal integer string=w576:string)  [unwired: 1 in]
                              n392 = Number To Decimal String(number=w572) -> (decimal integer string=w571:string)  [unwired: 1 in]
                              n393 = Concatenate Strings("WHERE CODE_ID =" ("condition"), w576, "AND DEVICE_ID = ", w571) -> (w584:string)
                              n394 = Bundle("RESULT"=w582, "result string"=w581) -> (w580:cluster{"RESULT":string, "result string":string})  [unwired: 1 in]
                              n395 = call <vilib>:"Clear Errors.vi"("error in (no error)"=w590) -> ("error out"=w589:errorcluster)  [unwired: 5 in, 1 out]
                              n396 = call <vilib>:"DB Tools Update Data.vi"("condition"=w584, "data"=w580, "error in (no error)"=w589, "columns"=w588, "table"=w591, "connection reference"=w579) -> ("error out"=w577:errorcluster, "connection reference out"=w578:T8)  [unwired: 4 in]
                            }
                          }
                        }
                        n397 = call <vilib>:"Simple Error Handler.vi"("error in (no error)"=w548) -> ()  [unwired: 4 in, 5 out]
                      }
                      frame #3 {
                        n398 = shared-variable "我的电脑\\180.lvlib\\备用1"(u16 0 ("备用1")) -> ()  [unwired: 1 in, 1 out]
                      }
                    }
                  }
                  frame 1000 {
                    n399 = stacked-sequence {
                      frame #0 {
                        w593 = "" ("传感器码")
                        n400 = shared-variable "我的电脑\\Global.lvlib\\传感器码"(w593) -> ()  [unwired: 1 in, 1 out]
                        n401 = local write "上管柱码"(w593) -> ()
                      }
                      frame #1 {
                        w596 = "请扫码！" ("通知内容")
                        n402 = call "浮动通知.vi"("通知内容"=w596) -> ()  [unwired: 11 in]
                        n403 = call "输入框.vi"("提示信息"=w596) -> ("条形码输出"=w594:string)
                        "上管柱码" <- w594
                        n404 = shared-variable "我的电脑\\Global.lvlib\\传感器码"(w594) -> ()  [unwired: 1 in, 1 out]
                        n405 = shared-variable "我的电脑\\180.lvlib\\备用1"(u16 1001 ("备用1")) -> ()  [unwired: 1 in, 1 out]
                      }
                    }
                  }
                  frame 1001 {
                    n406 = global read "Global1.vi" "联机模式"() -> (w597)
                    n407 = case shown="\"追溯\"" w597 {
                      frame "单机", Default {
                        n408 = shared-variable "我的电脑\\180.lvlib\\备用1"(u16 1002 ("备用1")) -> ()  [unwired: 1 in, 1 out]
                      }
                      frame "追溯" {
                        n409 = stacked-sequence {
                          frame #0 {
                            w600 = "'" ("字符串")
                            n410 = local read "上管柱码"() -> (w602:string)
                            n411 = local read "PRODUCTID"() -> (w599:string)
                            n412 = global read "Global1.vi" "联机模式"() -> (w619)
                            n413 = call "GetSQLstring.vi"("联机模式"=w619) -> ("错误输出"=w617:errorcluster, "连接字符串"=w618:string)  [unwired: 9 in]
                            n414 = Concatenate Strings("SELECT CODE_ID FROM CODE  WHERE CODE_MAIN= '" ("table"), w602, w600, " AND PRODUCT_ID='" ("字符串"), w599, w600) -> (w616:string)
                            n415 = call-poly <vilib>:"DB Tools Open Connection.vi"("error in (no error)"=w617, "connection information"=w618) -> ("error out"=w610:errorcluster, "connection reference"=w611:T8)  [unwired: 6 in]
                            n416 = call-poly <vilib>:"DB Tools Execute Query.vi"("error in (no error)"=w610, "SQL query"=w616, "connection reference"=w611) -> ("error out"=w614:errorcluster, "recordset reference"=w615:T12)  [unwired: 5 in]
                            n417 = call-poly <vilib>:"DB Tools Fetch Recordset Data.vi"("error in (no error)"=w614, "recordset reference"=w615) -> ("error out"=w608:errorcluster, "recordset data"=w613:variant[][])  [unwired: 3 in, 1 out]
                            n418 = Variant To Data(error in=w608, type=string[][] [], Variant=w613) -> (data=w607:string[][])  [unwired: 1 out]
                            n419 = Index Array(array=w607, index (row)=0 ("索引 (行)")) -> (element=w605:string[])  [unwired: 1 in]
                            n420 = Index Array(array=w605, index=0 ("索引 (行)")) -> (element=w603:string)
                            n421 = local write "CODE_ID"(w603) -> ()
                          }
                          frame #1 {
                            n422 = disable-structure shown="禁用" {
                              frame Disabled {
                                n423 = local read "前序deviceID"() -> ()  [unwired: 1 out]
                              }
                              frame Enabled {
                              }
                            }
                            n424 = global read "Global1.vi" "联机模式"() -> (w641)
                            n425 = local read "CODE_ID"() -> (w624:string)
                            n426 = call "GetSQLstring.vi"("联机模式"=w641) -> ("错误输出"=w639:errorcluster, "连接字符串"=w640:string)  [unwired: 9 in]
                            n427 = Concatenate Strings("SELECT RESULT_VALUE FROM RESULT  WHERE DEVICE_ID = \n" ("table"), "2" ("字符串"), " AND CODE_ID=" ("字符串"), w624) -> (w638:string)
                            n428 = call-poly <vilib>:"DB Tools Open Connection.vi"("error in (no error)"=w639, "connection information"=w640) -> ("error out"=w632:errorcluster, "connection reference"=w633:T8)  [unwired: 6 in]
                            n429 = call-poly <vilib>:"DB Tools Execute Query.vi"("error in (no error)"=w632, "SQL query"=w638, "connection reference"=w633) -> ("error out"=w636:errorcluster, "recordset reference"=w637:T12)  [unwired: 5 in]
                            n430 = call-poly <vilib>:"DB Tools Fetch Recordset Data.vi"("error in (no error)"=w636, "recordset reference"=w637) -> ("error out"=w630:errorcluster, "recordset data"=w635:variant[][])  [unwired: 3 in, 1 out]
                            n431 = Variant To Data(error in=w630, type=string[][] [], Variant=w635) -> (data=w626:string[][], error out=w623:errorcluster)
                            n432 = call <vilib>:"Clear Errors.vi"("error in (no error)"=w623) -> ("error out"=w622:errorcluster)  [unwired: 5 in, 1 out]
                            n433 = Index Array(array=w626, index (row)=0 ("索引 (行)")) -> (element=w628:string[])  [unwired: 1 in]
                            n434 = call <vilib>:"Simple Error Handler.vi"("error in (no error)"=w622) -> ()  [unwired: 4 in, 5 out]
                            n435 = Index Array(array=w628, index=0 ("索引 (行)")) -> (element=w625:string)
                            n436 = case shown="\"OK\"" w625 {
                              frame "假", Default {
                              }
                              frame "OK" {
                                n437 = shared-variable "我的电脑\\Global.lvlib\\传感器码"() -> (w644:string)  [unwired: 1 in, 1 out]
                                n438 = String Length(string=w644) -> (length=w645:i32)
                                n439 = Greater?(x=w645, y=4) -> (0:w643:bool)
                                n440 = case shown="真" w643 {
                                frame False {
                                }
                                frame True {
                                n441 = shared-variable "我的电脑\\180.lvlib\\备用1"(u16 1002 ("备用1")) -> ()  [unwired: 1 in, 1 out]
                                }
                                }
                              }
                              frame "NG" {
                              }
                            }
                          }
                        }
                      }
                    }
                  }
                }
              }
            }
          }
          event "删除": Value Change {
            n442 = event-data() -> ("NewVal"=w647:bool)  [unwired: 1 in, 5 out]
            n443 = case shown="真" w647 {
              tunnel: w648 -> [_ w650]
              frame False {
              }
              frame True {
                n444 = Concatenate Strings("确认删除“", "请选择要删除的产品", "”吗？") -> (w652:string)
                n445 = Two Button Dialog(message=w652) -> (T button?=w651:bool)  [unwired: 2 in]
                n446 = case shown="真" w651 {
                  tunnel: w650 -> [_ w656]
                  tunnel: "请选择要删除的产品" -> [_ w655]
                  frame False {
                  }
                  frame True {
                    n447 = call <vilib>:"Open Config Data.vi"("configuration file path"=w656) -> ("error out"=w658:errorcluster, "refnum"=w661:T3)  [unwired: 8 in, 1 out]
                    n448 = call <vilib>:"Remove Section.vi"("section"=w655, "error in (no error)"=w658, "refnum"=w661) -> ("error out"=w660:errorcluster, "section exists?"=w657:bool, "refnum out"=w659:T3)  [unwired: 6 in]
                    n449 = call <vilib>:"Close Config Data.vi"("error in (no error)"=w660, "refnum"=w659) -> ()  [unwired: 8 in, 2 out]
                    n450 = case shown="真" w657 {
                      frame False {
                        n451 = One Button Dialog(message="删除失败！\n请确认产品存在！" ("消息")) -> ()  [unwired: 1 in, 1 out]
                      }
                      frame True {
                        n452 = One Button Dialog(message="删除成功！" ("消息")) -> ()  [unwired: 1 in, 1 out]
                      }
                    }
                  }
                }
              }
            }
          }
          event "确定": Value Change {
            n453 = event-data() -> ("NewVal"=w664:bool)  [unwired: 1 in, 5 out]
            n454 = case shown="真" w664 {
              frame False {
              }
              frame True {
                n455 = stacked-sequence {
                  seq-local: [w666 _ _ _ _ _ _ _] -> [_ _ _ _ _ _ _ _]
                  frame #0 {
                    n456 = local read "产品型号"() -> (w665:string)
                    "产品型号" <- w665
                    n457 = shared-variable "我的电脑\\Global.lvlib\\产品型号"(w665) -> ()  [unwired: 1 in, 1 out]
                    n458 = String Subset(string=w665, offset (0)=u16 2 ("偏移量(0)"), length (rest)=u16 4 ("长度（剩余）")) -> (substring=w666:string)
                    n459 = Decimal String To Number(string=w666) -> ()  [unwired: 2 in, 2 out]
                  }
                  frame #1 {
                    n460 = local read "左工位坐标轴参数"() -> (w669:string[][])
                    n461 = Index Array(array=w669, index (row) #1=0 ("索引 (行)"), index (row) #2=1 ("索引 (行)"), index (row) #3=2 ("索引 (行)"), index (row) #4=3 ("索引 (行)")) -> (element #1=w685:string[], element #2=w680:string[], element #3=w679:string[], element #4=w678:string[])  [unwired: 4 in]
                    n462 = Index Array(array=w685, index=1 ("索引")) -> (element=w677:string)
                    n463 = Index Array(array=w680, index=1 ("索引")) -> (element=w675:string)
                    n464 = Index Array(array=w679, index=1 ("索引")) -> (element=w674:string)
                    n465 = Index Array(array=w678, index=1 ("索引")) -> (element=w673:string)
                    n466 = Fract/Exp String To Number(string=w677) -> (number=w676:dbl)  [unwired: 3 in, 1 out]
                    n467 = Fract/Exp String To Number(string=w675) -> (number=w672:dbl)  [unwired: 3 in, 1 out]
                    n468 = Fract/Exp String To Number(string=w674) -> (number=w671:dbl)  [unwired: 3 in, 1 out]
                    n469 = Fract/Exp String To Number(string=w673) -> (number=w670:dbl)  [unwired: 3 in, 1 out]
                    n470 = property on="力位移曲线" class="XYGraph (严格)"("XScale.Minimum"=w676) -> ()  [unwired: 2 in, 2 out]
                    n471 = property on="力位移曲线" class="XYGraph (严格)"("XScale.Maximum"=w672) -> ()  [unwired: 2 in, 2 out]
                    n472 = property on="力位移曲线" class="XYGraph (严格)"("YScale.Minimum"=w671) -> ()  [unwired: 2 in, 2 out]
                    n473 = property on="力位移曲线" class="XYGraph (严格)"("YScale.Maximum"=w670) -> ()  [unwired: 2 in, 2 out]
                  }
                  frame #2 {
                    n474 = local read "右工位坐标轴参数"() -> (w694:string[][])
                    n475 = Index Array(array=w694, index (row) #1=0 ("索引 (行)"), index (row) #2=1 ("索引 (行)"), index (row) #3=2 ("索引 (行)"), index (row) #4=3 ("索引 (行)")) -> (element #1=w706:string[], element #2=w701:string[], element #3=w700:string[], element #4=w699:string[])  [unwired: 4 in]
                    n476 = Index Array(array=w706, index=1 ("索引")) -> (element=w698:string)
                    n477 = Index Array(array=w701, index=1 ("索引")) -> (element=w697:string)
                    n478 = Index Array(array=w700, index=1 ("索引")) -> (element=w696:string)
                    n479 = Index Array(array=w699, index=1 ("索引")) -> (element=w695:string)
                    n480 = Fract/Exp String To Number(string=w698) -> (number=w693:dbl)  [unwired: 3 in, 1 out]
                    n481 = Fract/Exp String To Number(string=w697) -> (number=w692:dbl)  [unwired: 3 in, 1 out]
                    n482 = Fract/Exp String To Number(string=w696) -> (number=w691:dbl)  [unwired: 3 in, 1 out]
                    n483 = Fract/Exp String To Number(string=w695) -> (number=w690:dbl)  [unwired: 3 in, 1 out]
                    n484 = property on="力位移曲线 2" class="XYGraph (严格)"("XScale.Minimum"=w693) -> ()  [unwired: 2 in, 2 out]
                    n485 = property on="力位移曲线 2" class="XYGraph (严格)"("XScale.Maximum"=w692) -> ()  [unwired: 2 in, 2 out]
                    n486 = property on="力位移曲线 2" class="XYGraph (严格)"("YScale.Minimum"=w691) -> ()  [unwired: 2 in, 2 out]
                    n487 = property on="力位移曲线 2" class="XYGraph (严格)"("YScale.Maximum"=w690) -> ()  [unwired: 2 in, 2 out]
                  }
                  frame #3 {
                    n488 = local read "左工位判定框参数"() -> (w720:string[][])
                    n489 = Index Array(array=w720, index (row) #1=0 ("索引 (行)"), index (row) #2=1 ("索引 (行)"), index (row) #3=2 ("索引 (行)"), index (row) #4=3 ("索引 (行)")) -> (element #1=w728:string[], element #2=w723:string[], element #3=w722:string[], element #4=w721:string[])  [unwired: 4 in]
                    n490 = Index Array(array=w723, index=1 ("索引")) -> (element=w714:string)
                    n491 = Index Array(array=w728, index=1 ("索引")) -> (element=w715:string)
                    n492 = Index Array(array=w721, index=1 ("索引")) -> (element=w712:string)
                    n493 = Index Array(array=w722, index=1 ("索引")) -> (element=w713:string)
                    n494 = local read "力位移曲线"() -> (w733:cluster{dbl[], dbl[]}[])
                    n495 = Fract/Exp String To Number(string=w714) -> (number=w718:dbl)  [unwired: 3 in, 1 out]
                    n496 = Fract/Exp String To Number(string=w715) -> (number=w719:dbl)  [unwired: 3 in, 1 out]
                    n497 = Fract/Exp String To Number(string=w712) -> (number=w717:dbl)  [unwired: 3 in, 1 out]
                    n498 = Fract/Exp String To Number(string=w713) -> (number=w716:dbl)  [unwired: 3 in, 1 out]
                    n499 = for {
                      tunnel: [w740] -> w711 mode=indexing
                      tunnel: w733 -> [w739] mode=indexing
                      tunnel: w719 -> [w737]
                      tunnel: w718 -> [w736]
                      tunnel: w717 -> [w735]
                      tunnel: w716 -> [w734]
                      i -> [w738]
                      n500 = case shown="0" w738 {
                        tunnel: [w741 w746] -> w740
                        tunnel: w739 -> [w741 _]
                        tunnel: w737 -> [_ w745]
                        tunnel: w736 -> [_ w744]
                        tunnel: w735 -> [_ w743]
                        tunnel: w734 -> [_ w742]
                        frame Default {
                        }
                        frame 0 {
                          n501 = Build Array(w745, w745, w744, w744, w745) -> (w747:dbl[])
                          n502 = Build Array(w742, w743, w743, w742, w742) -> (w748:dbl[])
                          n503 = Bundle(w747, w748) -> (w746:cluster{dbl[], dbl[]})  [unwired: 1 in]
                        }
                      }
                    }
                    n504 = local write "力位移曲线"(w711) -> ()
                  }
                  frame #4 {
                    n505 = local read "右工位判定框参数"() -> (w749:string[][])
                    n506 = Index Array(array=w749, index (row) #1=0 ("索引 (行)"), index (row) #2=1 ("索引 (行)"), index (row) #3=2 ("索引 (行)"), index (row) #4=3 ("索引 (行)")) -> (element #1=w767:string[], element #2=w762:string[], element #3=w761:string[], element #4=w760:string[])  [unwired: 4 in]
                    n507 = Index Array(array=w762, index=1 ("索引")) -> (element=w754:string)
                    n508 = Index Array(array=w767, index=1 ("索引")) -> (element=w755:string)
                    n509 = Index Array(array=w760, index=1 ("索引")) -> (element=w752:string)
                    n510 = Index Array(array=w761, index=1 ("索引")) -> (element=w753:string)
                    n511 = local read "力位移曲线 2"() -> (w750:cluster{dbl[], dbl[]}[])
                    n512 = Fract/Exp String To Number(string=w754) -> (number=w758:dbl)  [unwired: 3 in, 1 out]
                    n513 = Fract/Exp String To Number(string=w755) -> (number=w759:dbl)  [unwired: 3 in, 1 out]
                    n514 = Fract/Exp String To Number(string=w752) -> (number=w757:dbl)  [unwired: 3 in, 1 out]
                    n515 = Fract/Exp String To Number(string=w753) -> (number=w756:dbl)  [unwired: 3 in, 1 out]
                    n516 = for {
                      tunnel: [w778] -> w751 mode=indexing
                      tunnel: w750 -> [w777] mode=indexing
                      tunnel: w759 -> [w775]
                      tunnel: w758 -> [w774]
                      tunnel: w757 -> [w773]
                      tunnel: w756 -> [w772]
                      i -> [w776]
                      n517 = case shown="0" w776 {
                        tunnel: [w779 w784] -> w778
                        tunnel: w777 -> [w779 _]
                        tunnel: w775 -> [_ w783]
                        tunnel: w774 -> [_ w782]
                        tunnel: w773 -> [_ w781]
                        tunnel: w772 -> [_ w780]
                        frame Default {
                        }
                        frame 0 {
                          n518 = Build Array(w783, w783, w782, w782, w783) -> (w785:dbl[])
                          n519 = Build Array(w780, w781, w781, w780, w780) -> (w786:dbl[])
                          n520 = Bundle(w785, w786) -> (w784:cluster{dbl[], dbl[]})  [unwired: 1 in]
                        }
                      }
                    }
                    n521 = local write "力位移曲线 2"(w751) -> ()
                  }
                  frame #5 {
                    n522 = global read "Global1.vi" "联机模式"() -> (w787)
                    n523 = case shown="\"追溯\"" w787 {
                      frame "单机", Default {
                      }
                      frame "追溯" {
                        n524 = local read "产品型号"() -> (w788:string)
                        n525 = call "GET_PRODUCT_ID.vi"("PRODFUCT_NAME"=w788) -> ("PRODUCT_ID"=w790:string)  [unwired: 10 in]
                        n526 = call "查询前序设备.vi"("PRODUCT_ID"=w790) -> ("前序工位"=w789:string[])  [unwired: 10 in]
                        n527 = call "Get_Device_ID.vi"() -> ("Device_ID"=w793:string)  [unwired: 10 in, 1 out]
                        n528 = Index Array(array=w789, index=0 ("索引")) -> (element=w792:string)
                        n529 = local write "deviceID"(w793) -> ()
                        n530 = local write "PRODUCTID"(w790) -> ()
                        n531 = local write "前序deviceID"(w792) -> ()
                      }
                    }
                  }
                  frame #6 {
                    n532 = global read "Global1.vi" "联机模式"() -> (w794)
                    n533 = case shown="\"追溯\"" w794 {
                      tunnel: w794 -> [_ w813]
                      frame "单机", Default {
                      }
                      frame "追溯" {
                        n534 = local read "用户名"() -> (w796:string)
                        n535 = call "GetSQLstring.vi"("联机模式"=w813) -> ("错误输出"=w811:errorcluster, "连接字符串"=w812:string)  [unwired: 9 in]
                        n536 = Concatenate Strings("SELECT USER_ID FROM [User]  WHERE USER_NAME ='" ("字符串"), w796, "'" ("字符串")) -> (w810:string)
                        n537 = call-poly <vilib>:"DB Tools Open Connection.vi"("error in (no error)"=w811, "connection information"=w812) -> ("error out"=w804:errorcluster, "connection reference"=w805:T8)  [unwired: 6 in]
                        n538 = call-poly <vilib>:"DB Tools Execute Query.vi"("error in (no error)"=w804, "SQL query"=w810, "connection reference"=w805) -> ("error out"=w808:errorcluster, "recordset reference"=w809:T12)  [unwired: 5 in]
                        n539 = call-poly <vilib>:"DB Tools Fetch Recordset Data.vi"("error in (no error)"=w808, "recordset reference"=w809) -> ("error out"=w802:errorcluster, "recordset data"=w807:variant[][])  [unwired: 3 in, 1 out]
                        n540 = Variant To Data(error in=w802, type=string[][] [], Variant=w807) -> (data=w801:string[][])  [unwired: 1 out]
                        n541 = Index Array(array=w801, index (row)=0 ("索引 (行)")) -> (element=w799:string[])  [unwired: 1 in]
                        n542 = Index Array(array=w799, index=0 ("索引 (行)")) -> (element=w797:string)
                        n543 = local write "USERID"(w797) -> ()
                      }
                    }
                  }
                  frame #7 {
                    w814 = "参数装载成功！" ("消息")
                    n544 = call "浮动通知.vi"("通知内容"=w814) -> ()  [unwired: 11 in]
                    n545 = One Button Dialog(message=w814) -> ()  [unwired: 1 in, 1 out]
                  }
                }
              }
            }
          }
          event "添加": Value Change {
            n546 = event-data() -> ("NewVal"=w817:bool)  [unwired: 1 in, 5 out]
            n547 = local read "请输入添加的产品名称"() -> (w818:string)
            n548 = call <vilib>:"Trim Whitespace.vi"("string"=w818) -> ("trimmed string"=w819:string)  [unwired: 1 in]
            n549 = White Space?(1:w819) -> (0:w820:bool)
            n550 = case shown="假" w820 {
              tunnel: w815 -> [w823 _]
              tunnel: w817 -> [w822 _]
              tunnel: w816 -> [w821 _]
              frame False {
                n551 = case shown="真" w822 {
                  tunnel: w823 -> [_ w825]
                  tunnel: w821 -> [_ w824]
                  frame False {
                  }
                  frame True {
                    n552 = for {
                      tunnel: w825 -> [w828] mode=indexing
                      tunnel: w824 -> [w827]
                      n553 = call "Read_Write ParaINI File.vi"("Mode"=enum16{"Read", "Write"}."Write", "Section"="请输入添加的产品名称", "Filepath"=w827, "Ctl Refnum"=w828) -> ()  [unwired: 7 in, 1 out]
                    }
                  }
                }
              }
              frame True {
                w830 = 64 items=["None"=0, "Hand, Error, Stop"=16, "Question"=32, "Exclamation, Warning"=48, "Asterisk, Information"=64] ("icon")
                w831 = 0 items=["OK", "OKCancel", "AbortRetryIgnore", "YesNoCancel", "YesNo", "RetryCancel"] ("buttons")
                n554 = call "信息框（标题、文本、图标）.vi"("icon"=w830, "buttons"=w831, "caption"="添加失败", "text"="请输入产品名称!") -> ()  [unwired: 6 in, 2 out]
              }
            }
          }
          event "产品型号": Value Change {
            n555 = event-data() -> ()  [unwired: 1 in, 6 out]
            n556 = stacked-sequence {
              tunnel: w834 -> [_ w837]
              tunnel: w835 -> [_ w836]
              frame #0 {
              }
              frame #1 {
                n557 = for {
                  tunnel: w837 -> [w840] mode=indexing
                  tunnel: w836 -> [w839]
                  n558 = local read "产品型号"() -> (w838:string)
                  n559 = call "Read_Write ParaINI File.vi"("Mode"=enum16{"Read", "Write"}."Read", "Section"=w838, "Filepath"=w839, "Ctl Refnum"=w840) -> ()  [unwired: 7 in, 1 out]
                }
              }
            }
          }
          event "退出": Value Change {
            n560 = event-data() -> ()  [unwired: 1 in, 6 out]
            n561 = control-ref of="本VI"() -> (w847:refnum<vi>)
            n562 = invoke class="VI" method="FP.Close"(reference=w847) -> (reference out=w845:refnum<vi>, error out=w846:errorcluster)  [unwired: 2 in, 1 out]
            n563 = Close Reference(reference=w845, error in (no error)=w846) -> ()  [unwired: 1 out]
            n564 = vi-ref "client.vi"() -> (w842:refnum<vi>)
            n565 = invoke class="VI" method="FP.Close"(reference=w842) -> (reference out=w843:refnum<vi>, error out=w844:errorcluster)  [unwired: 2 in, 1 out]
            n566 = Close Reference(reference=w843, error in (no error)=w844) -> ()  [unwired: 1 out]
            n567 = global write "Global.vi" "程序关闭"(TRUE ("程序关闭")) -> ()
          }
          event "更新": Value Change {
            n568 = event-data() -> ("NewVal"=w851:bool)  [unwired: 1 in, 5 out]
            n569 = case shown="真" w851 {
              tunnel: w850 -> [_ w854]
              tunnel: w849 -> [_ w853]
              frame False {
              }
              frame True {
                n570 = for {
                  tunnel: w854 -> [w859]
                  tunnel: w853 -> [w858] mode=indexing
                  tunnel: [w857] -> w852
                  n571 = local read "产品型号"() -> (w861:string)
                  n572 = call "Read_Write ParaINI File.vi"("Mode"=enum16{"Read", "Write"}."Write", "Section"=w861, "Filepath"=w859, "Ctl Refnum"=w858) -> ("error out"=w857:errorcluster)  [unwired: 7 in]
                }
                n573 = case shown="无错误" w852 {
                  frame No Error {
                    n574 = call "浮动通知.vi"("通知内容"="更新成功！") -> ()  [unwired: 11 in]
                  }
                  frame Error {
                    n575 = call "浮动通知.vi"("通知内容"="更新失败！") -> ()  [unwired: 11 in]
                  }
                }
              }
            }
          }
          event "请输入添加的产品名称": Value Change {
            n576 = event-data() -> ("NewVal"=w862:string)  [unwired: 1 in, 5 out]
            n577 = control-ref of="产品型号"() -> (w863:refnum<vi>)
            n578 = property on="属性节点" class="CmbBox"(reference=w863) -> ("Strings[]"=w864:string[])  [unwired: 1 in, 2 out]
            n579 = for {
              tunnel: w862 -> [w865]
              tunnel: w864 -> [w866] mode=indexing
              n580 = Equal?(x=w865, y=w866) -> (x = y?=w867:bool)
              n581 = case shown="真" w867 {
                tunnel: w865 -> [_ w868]
                frame False {
                }
                frame True {
                  n582 = stacked-sequence {
                    tunnel: w868 -> [w874 _]
                    frame #0 {
                      w869 = 64 items=["None"=0, "Hand, Error, Stop"=16, "Question"=32, "Exclamation, Warning"=48, "Asterisk, Information"=64] ("icon")
                      w870 = 0 items=["OK", "OKCancel", "AbortRetryIgnore", "YesNoCancel", "YesNo", "RetryCancel"] ("buttons")
                      n583 = Concatenate Strings("已经存在产品”" ("text"), w874, "“\n请勿重复添加！" ("字符串")) -> (w872:string)
                      n584 = call "信息框（标题、文本、图标）.vi"("icon"=w869, "buttons"=w870, "caption"="产品重复", "text"=w872) -> ()  [unwired: 6 in, 2 out]
                    }
                    frame #1 {
                      n585 = local write "请输入添加的产品名称"("" ("请输入添加的产品名称")) -> ()
                    }
                  }
                }
              }
            }
          }
          event Panel Close? {
            n586 = event-data() -> ()  [unwired: 1 in, 4 out]
            n587 = global write "Global.vi" "程序关闭"(TRUE ("程序关闭")) -> ()
            n588 = control-ref of="本VI"() -> (w882:refnum<vi>)
            n589 = invoke class="VI" method="FP.Close"(reference=w882) -> (reference out=w880:refnum<vi>, error out=w881:errorcluster)  [unwired: 2 in, 1 out]
            n590 = Close Reference(reference=w880, error in (no error)=w881) -> ()  [unwired: 1 out]
            n591 = vi-ref "client.vi"() -> (w877:refnum<vi>)
            n592 = invoke class="VI" method="FP.Close"(reference=w877) -> (reference out=w878:refnum<vi>, error out=w879:errorcluster)  [unwired: 2 in, 1 out]
            n593 = Close Reference(reference=w878, error in (no error)=w879) -> ()  [unwired: 1 out]
            n594 = event-data("Discard?"=TRUE ("放弃？")) -> ()  [unwired: 1 in, 1 out]
          }
          event "确定按钮": Value Change {
            n595 = event-data() -> ()  [unwired: 1 in, 6 out]
            n596 = vi-ref "User_manager.vi"() -> (w886:refnum<vi>)
            n597 = call "CallVI.vi"("VI引用"=w886, "状态"=T1."Maximized") -> ()  [unwired: 11 in, 3 out]
          }
          event "设备故障": Value Change {
            n598 = event-data() -> ()  [unwired: 1 in, 6 out]
            n599 = global read "Global1.vi" "用户信息"() -> (w892)
            n600 = Unbundle By Name(w892) -> ("用户名"=w890)
            n601 = Bundle("设备名称"="上下管柱总成装配", "用户名"=w890, "设备状态"="设备状态", "附加信息"="附加信息") -> (w887:T2)  [unwired: 1 in]
            n602 = vi-ref "client.vi"() -> (w894:refnum<vi>)
            n603 = invoke class="VI" method="Ctrl Val.Set"(reference=w894, "Control Name"="设备信息" ("控件名"), "Value"=w887) -> ()  [unwired: 2 in, 5 out]
          }
          event "设备缺料": Value Change {
            n604 = event-data() -> ()  [unwired: 1 in, 6 out]
            n605 = global read "Global1.vi" "用户信息"() -> (w900)
            n606 = Unbundle By Name(w900) -> ("用户名"=w898)
            n607 = Bundle("设备名称"="上下管柱总成装配", "用户名"=w898, "设备状态 2"="设备状态 2", "附加信息 2"="附加信息 2") -> (w895:T13)  [unwired: 1 in]
            n608 = vi-ref "client.vi"() -> (w902:refnum<vi>)
            n609 = invoke class="VI" method="Ctrl Val.Set"(reference=w902, "Control Name"="设备信息" ("控件名"), "Value"=w895) -> ()  [unwired: 2 in, 5 out]
          }
          event "质量报警": Value Change {
            n610 = event-data() -> ()  [unwired: 1 in, 6 out]
            n611 = global read "Global1.vi" "用户信息"() -> (w908)
            n612 = Unbundle By Name(w908) -> ("用户名"=w906)
            n613 = Bundle("设备名称"="上下管柱总成装配", "用户名"=w906, "设备状态 3"="设备状态 3", "附加信息 3"="附加信息 3") -> (w903:T14)  [unwired: 1 in]
            n614 = vi-ref "client.vi"() -> (w910:refnum<vi>)
            n615 = invoke class="VI" method="Ctrl Val.Set"(reference=w910, "Control Name"="设备信息" ("控件名"), "Value"=w903) -> ()  [unwired: 2 in, 5 out]
          }
        }
        n616 = global read "Global.vi" "程序关闭"() -> (w113:bool)
      }
    }
    frame #3 {
      n617 = global write "Global.vi" "程序关闭"(TRUE ("程序关闭")) -> ()
    }
  }
